vi "SEC code V4.9.vi"() -> ()   [LabVIEW 2022 SP3]
uses:
  SEC code V3.1/Drivers and Aux files/user.lib/atmcd32d.llb/Shutter_type typedef.ctl
  C:/Program Files/Metrohm Autolab/Autolab SDK 1.10/EcoChemie.Autolab.Sdk.dll
  Program Files/Metrohm Autolab/Autolab SDK 1.10/EcoChemie.Autolab.Sdk.dll
  SEC code V3.1/Drivers and Aux files/State.ctl
  SEC code V3.1/Drivers and Aux files/SECenumctl.ctl
  SEC code V3.1/Drivers and Aux files/user.lib/atmcd32d.llb/TriggerMode_mode typedef.ctl
  SEC code V3.1/Drivers and Aux files/OSSPEC.ctl
  SEC code V3.1/Drivers and Aux files/OSPEC-enum.ctl
  Labview/IVIUM/IVIUM_remdriver.lvlib
panel:
  out "POtential PD":dbl
  out "Current PD":dbl
  in  "Tab Control 5":enum32{"AUTOLAB", "IVIUM", "iDUS", "Kymera"}(tab)
  out "current":dbl
  out "Error after autolab connection?":errorcluster
  out "Autolab Connected?":bool
  out "Voltage":dbl
  out "PotentialOverload":bool
  out "Bandwidth":i32(ring) items=["UltraHigh_Speed", "High_Speed", "High_Stability"]
  out "CurrentRange":i32(ring) items=["CR07_1A"=0, "CR06_10A"=1, "CR01_100A"=2, "CR00_1000A"=3, "CR05_20A"=20, "CR04_40A"=40, "CR03_50A"=60, "CR02_80A"=80, "CR19_1pA"=-12, "CR18_10pA"=-11, "CR17_100pA"=-10, "CR16_1nA"=-9, "CR15_10nA"=-8, "CR14_100nA"=-7, "CR13_1uA"=-6, "CR12_10uA"=-5, "CR11_100uA"=-4, "CR10_1mA"=-3, "CR09_10mA"=-2, "CR08_100mA"=-1]
  out "Mode":i32(ring) items=["Potentiostatic", "Galvanostatic"]
  out "Measured voltage":dbl
  out "CurrentOverload":bool
  out "Cell on?":bool
  out "current":dbl caption="Current (A)" format="%_4g"
  out "cell on":bool
  out "V (during measurment)":dbl
  out "Potentiostat Status":string
  out "T reached?":bool
  out "Shut down sequence run?":bool
  out "Curent Temp":i32
  in  "Tab Control 4":T1(tab)
  in  "Use autolab?":bool=TRUE
  in  "Embedded Exe File":path=path "C:/Program Files/Metrohm Autolab/Autolab SDK 2.1/Hardware Setup Files/Adk.x"
  in  "Hardware Setup File":path=path "C:/ProgramData/Metrohm Autolab/13.0/HardwareSetup.AUT55157.xml"
  in  "Bandwidth 2":i32(ring)=2 items=["UltraHigh_Speed", "High_Speed", "High_Stability"]
  in  "Start potential (V)":dbl=0.2
  in  "Stop potential (V)":dbl=0.7
  in  "Increment (V)":dbl=0.05
  in  "Default Potential (V)":dbl=0.2
  in  "Wait before \nspectrum (s)":dbl=0.1
  in  "Equilibration \ntime (s)":u32=5
  in  "Reverse Scan\ndirection":bool
  in  "(update and read)":bool
  in  "Tab Control 3":T2(tab)
  in  "Inetegration Time (us)":i32=5000
  in  "Continuous \nStrobe Delay (us)":i32
  in  "Use iDus?":bool=TRUE
  in  "Return detector \nto room T?":bool
  in  "Init, Cool, read dark,\nOR\nWarm/de-init detector":bool
  in  "Temperature\n(degrees C)":i32=-80
  in  "Number of scans in kinetic cycle":i32=30
  in  "Exposure time (s)":dbl=0.03
  in  "Tab Control 2":T3(tab)
  in  "V 1 time (s)":dbl=10.0
  in  "V off time":dbl=30.0
  in  "Sampling delay (s)":dbl
  in  "V 2 time (s)":dbl=20.0
  in  "Run OSPSEC":bool
  in  "squre wave":bool
  out "OCP I (close to 0)":dbl
  out "OCP":dbl format="%_3f"
  in  "V1 (V)":dbl=0.4
  in  "V2 (V)":dbl=0.8
  in  "Slow sample time (s)":dbl=1500.0
  out "Time during PD":u32
  in  "File Name":string="test-1"
  in  "Path":path=path "C:/Data"
  in  "Tab Control":T4(tab)
  out "?":T5(graph)
  out "?":cluster{i32[], dbl[]}(graph)
  out "?":T5(graph)
  out "?":T5(graph)
  out "?":cluster{dbl[], dbl[]}(graph)
  out "?":cluster{i32[], "array":i32[]}(graph)
  out "I_overload":bool
  out "Aninput1_overload":bool
  out "E_overload":bool
  out "cell-off button pressed":bool
  in  "Default\nCurrent range":T6(ring)=enum."100 uA"
  in  "Default Filter":T7(ring)=enum."10 kHz"
  out "Device serial number":string
  in  "Set Stability":T8(ring)=enum."Standard"
  out "Number of Spectrometers":i32
  out "IDus not in read loop? (kinetic)":bool
  out "Get status return code":dbl
  out "xpixels":i32
  out "ypixels":i32
  out "Calculated exposure time":sgl format="%.2f"
  out "Check timings return code":u32
  out "Set temprature\nreturn code":u32
  out "get aquired data return code":u32
  out "Start Aquisition return code":u32
  out "Init. return code":u32
  out "Cooler Off return code":u32
  out "Time before the start of current aquisition (ms)":u32
  out "Time  after the aquisition (before fetch data), (ms)":u32
  in  "Shutter opens on TTL":T9=enum."TTL High"
  in  "Shutter open and close time":i32
  out "Get aqisition ok? (kinetic mode)":bool
  out "Time taken to apply V2":u32
  out "Values to re-intialise to at end\nof the measument":T10
  out "V2 applied?":bool
  out "ContinuousStrobe Out":u32
  out "Wrapper Out":u32
  out "WL Values":dbl[](array[numeric])
  out "Adc":refnum<k24>
  out "Sampler 2":refnum<k24>
  out "Dio":refnum<k24>
  out "Dac":refnum<k24>
  out "instrument":refnum<k24>
  out "Ei":refnum<k24>
  out "AutolabConnection":refnum<k24>
  out "EI status supported for":string[](array[string])
  out "TemperatureOverload":bool
  out "ManualCellSwitch":bool
  out "Oscillation":bool
  in  "Exit and disconnect":bool
  # "Checklist for avoiding errors:\n(1) Light on the IVIUM should be blue with red flashes\nIf the system crahes and the light is red then connect and disconnect in IVUM soft/turn stat off/on\n(2) Maya Pro should read in ocean view/or the get intensity program\nIf maya is not reading connect and disconnect USB\n(3) If errors persist rrepeat steps 1 + 2 then re-compile code by clicking the\nwhite (run) whilst holding down CRTL + (left) SHIFT\n(4) At the end of a potential decay measurment click exit before starting a new measurment\n(5) IF USING THE iDus DO NOT EXIT WITHOUT WARMING CAMERA BACK TO ROOM T,YOU \nWILL DAMAGE IT \n(6) if the IVIUM.dll does not load click broken arrows and \"show error\" until you see the call library function (see blue circles). Double click on this and paste the following into the directory (red circle):   \n%windir%\\Labview\\IVIUM\\IVIUM_remdriver.dll"
  # "Program control"
  # "Potential decay control"
  # "Spectrometer control"
  # "System status"
  # "SEC control"
  # "Cell on?"
  # "Use the integration time program in the same folder as this program\nto get the optimum value. For kinetic mode the time resolution is limited \nby integration time"
  # "Unless you know what you are doing keep these at 0.03 and 30"
  # "I overload overload"
  # "off button pressed"
  # "Aninput1 overload"
  # "E overload"
  # "OSPEC loop exit"
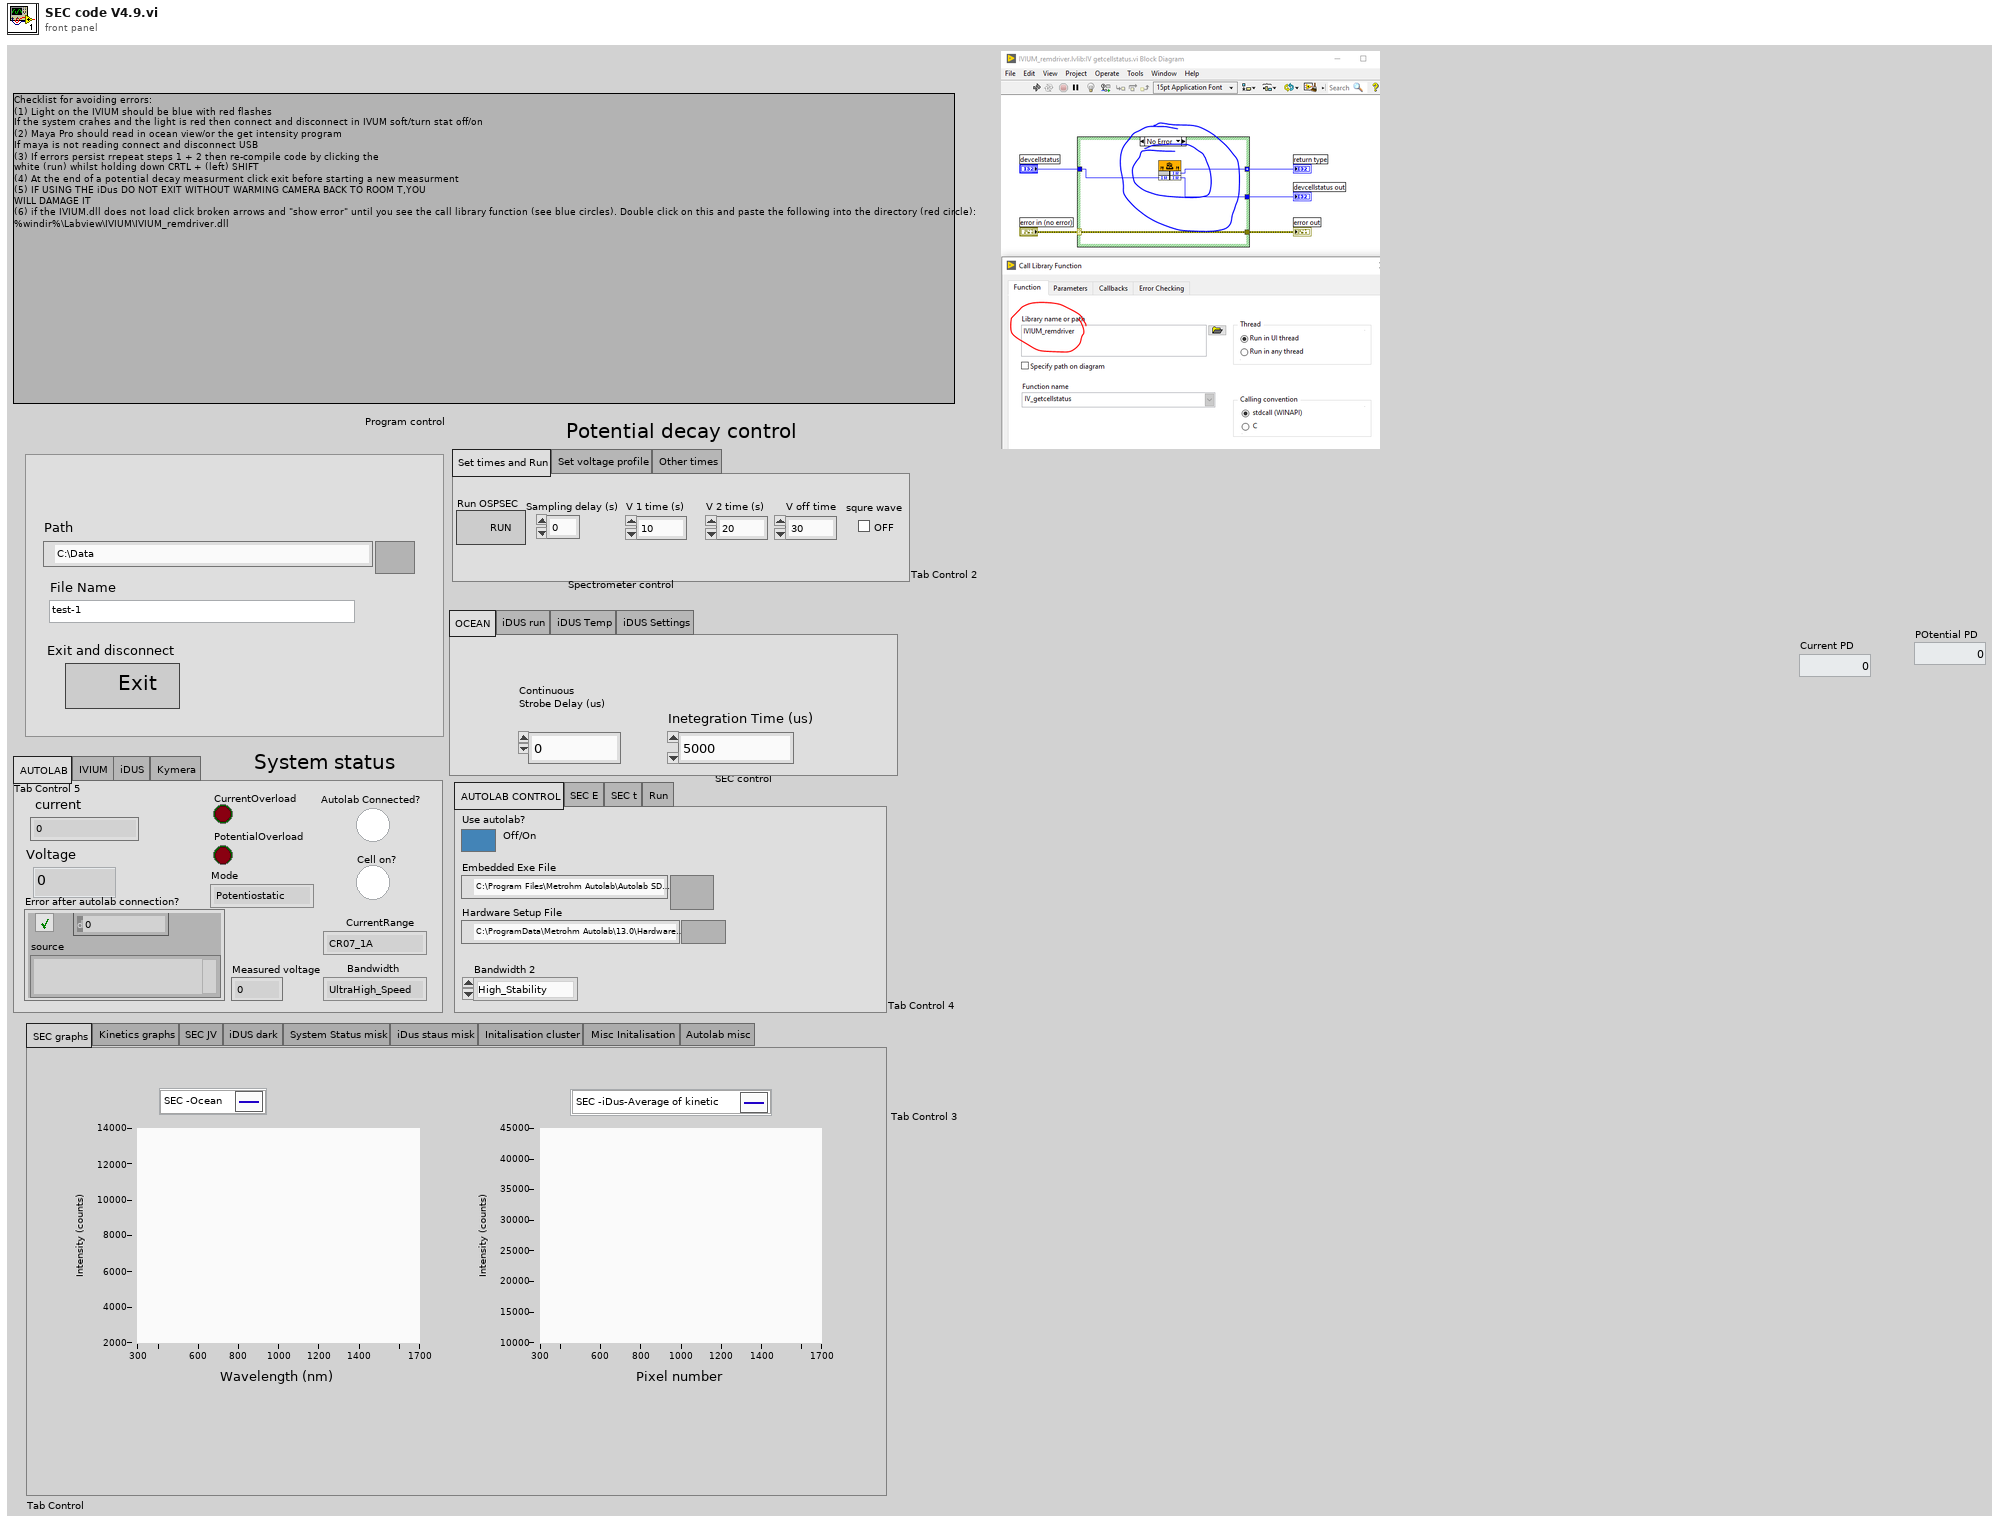
[diagram p1: front panel]
types:
  T1 = enum32{"AUTOLAB CONTROL", "SEC E", "SEC t", "Run"}
  T2 = enum32{"OCEAN", "iDUS run", "iDUS Temp", "iDUS Settings"}
  T3 = enum32{"Set times and Run", "Set voltage profile", "Other times"}
  T4 = enum32{"SEC graphs", "Kinetics graphs", "SEC JV", "iDUS dark", "System Status misk", "iDus staus misk", "Initalisation cluster", "Misc Initalisation ", "Autolab misc"}
  T5 = cluster{"WL Values":dbl[], "Spectrum Values":dbl[]}
  T6 = enum16{"10 A", "1 A", "100 mA", "10 mA", "1 mA", "100 uA", "10 uA", "1 uA", "100 nA", "10 nA", "1 nA", "100 pA", "10 pA", "1 pA"}
  T7 = enum16{"1 MHz", "100 kHz", "10 kHz", "1 kHz", "10 Hz"}
  T8 = enum16{"High Speed", "Standard", "High Stability"}
  T9 = typedef "Shutter_type typedef.ctl" = enum16{"TTL Low", "TTL High"}
  T10 = cluster{"Currents":dbl[], "Potentials":dbl[], "Device Status":string, "Device serial no":string, "Current":dbl, "Default \nPotential":dbl, "I overload":bool, "Cell On":bool, "E overload":bool, "Aninput1 overload":bool, "Cell off button pressed":bool, "Start potential":dbl, "Stop potential":dbl, "Increment":dbl, "SEC":dbl[], "Path":path, "File name":string}
  T11 = cluster{"Current array":dbl[], "Potential array":dbl[], "Status":string, "Serial No":string, "Current":dbl, "Default\n potential":dbl, "I overload":bool, "Cell on":bool, "E overload":bool, "Cell of button pressed":bool, "Aninput1 overload":bool, "Stop \npotential":dbl, "Start \npotential":dbl, "Increment":dbl, "Spectrum":dbl[][], "Path":path, "File Name":string, "Sample rate":dbl, "V2 time":dbl, "V off time":dbl, "V 2":dbl, "V 1":dbl, "V1 time":dbl, "Time array":dbl[], "Integration time":i32, "Continous strobe delay":i32, "Time elapsed ":i32, "Start time":i32, "Time for E measurment":i32[], "Time for I measurment ":i32[], "Time for spectrum measurment":i32[], "Return detector to \nroom T":bool, "Number of scans in kinetic cycle":i32, "Exposure time":i32}
  T12 = typedef "State.ctl" = enum16{"Initialize", "Wait for Event", "Run SEC", "Run OSPEC", "Initialse and cool iDus", "Exit"}
  T13 = typedef "SECenumctl.ctl" = enum16{"Read spectrum from Ocean", "Read spectrum from iDus", "Apply potential", "Wait", "Apply potential Autolab"}
  T14 = typedef "TriggerMode_mode typedef.ctl" = enum16{"Internal", "External", "N/A (2)", "N/A (3)", "N/A (4)", "N/A (5)", "External Start", "External Exposure (Bulb)", "N/A (8)", "External FVB EM", "Software", "N/A (11)", "External Charge Shifting"}
  T15 = typedef "OSSPEC.ctl" = enum16{"Read Potential and spectrum", "Read current and spectrum", "Reinitialise Cell", "Apply V1", "End measurment", "Apply V2"}
  T16 = typedef "OSPEC-enum.ctl" = enum16{"Check exit", "Read", "Wait"}
  T17 = enum16{"off", "EStat4EL", "EStat2EL", "EStatDummy1", "EStatDummy2", "EStatDummy3", "EStatDummy4", "IStat4EL", "IStat2EL", "IStatDummy", "BiStat4EL", "BiStat2EL"}
  T18 = typedef "Error Code Enum typedef.ctl" = enum32{"N/A (0)", "DRV_ERROR_CODES", "DRV_SUCCESS", "DRV_VXDNOTINSTALLED", "DRV_ERROR_SCAN", "DRV_ERROR_CHECK_SUM", "DRV_ERROR_FILELOAD", "DRV_UNKNOWN_FUNC", "DRV_ERROR_VXD_INIT", "DRV_ERROR_ADDRESS", "DRV_ERROR_PAGELOCK", "DRV_ERROR_PAGEUNLOCK", "DRV_ERROR_BOARDTEST", "DRV_ERROR_ACK", "DRV_ERROR_UP_FIFO", "DRV_ERROR_PATTERN", "N/A (16)", "DRV_ACQUISITION_ERRORS", "DRV_ACQ_BUFFER", "DRV_ACQ_DOWNFIFO_FULL", "DRV_PROC_UNKONWN_INSTRUCTION", "DRV_ILLEGAL_OP_CODE", "DRV_KINETIC_TIME_NOT_MET", "DRV_ACCUM_TIME_NOT_MET", "DRV_NO_NEW_DATA", "N/A (25)", "DRV_SPOOLERROR", "N/A (27)", "N/A (28)", "N/A (29)", "N/A (30)", "N/A (31)", "N/A (32)", "DRV_TEMPERATURE_CODES", "DRV_TEMPERATURE_OFF", "DRV_TEMPERATURE_NOT_STABILIZED", "DRV_TEMPERATURE_STABILIZED", "DRV_TEMPERATURE_NOT_REACHED", "DRV_TEMPERATURE_OUT_RANGE", "DRV_TEMPERATURE_NOT_SUPPORTED", "DRV_TEMPERATURE_DRIFT", "N/A (41)", "N/A (42)", "N/A (43)", "N/A (44)", "N/A (45)", "N/A (46)", "N/A (47)", "N/A (48)", "DRV_GENERAL_ERRORS", "DRV_INVALID_AUX", "DRV_COF_NOTLOADED", "DRV_FPGAPROG", "DRV_FLEXERROR", "DRV_GPIBERROR", "N/A (55)", "N/A (56)", "N/A (57)", "N/A (58)", "N/A (59)", "N/A (60)", "N/A (61)", "N/A (62)", "N/A (63)", "DRV_DATATYPE", "DRV_DRIVER_ERRORS", "DRV_P1INVALID", "DRV_P2INVALID", "DRV_P3INVALID", "DRV_P4INVALID", "DRV_INIERROR", "DRV_COFERROR", "DRV_ACQUIRING", "DRV_IDLE", "DRV_TEMPCYCLE", "DRV_NOT_INITIALIZED", "DRV_P5INVALID", "DRV_P6INVALID", "DRV_INVALID_MODE", "DRV_INVALID_FILTER", "DRV_I2CERRORS", "DRV_I2CDEVNOTFOUND", "DRV_I2CTIMEOUT", "DRV_P7INVALID", "N/A (84)", "N/A (85)", "N/A (86)", "N/A (87)", "N/A (88)", "N/A (89)", "DRV_IOCERROR", "DRV_VRMVERSIONERROR"}
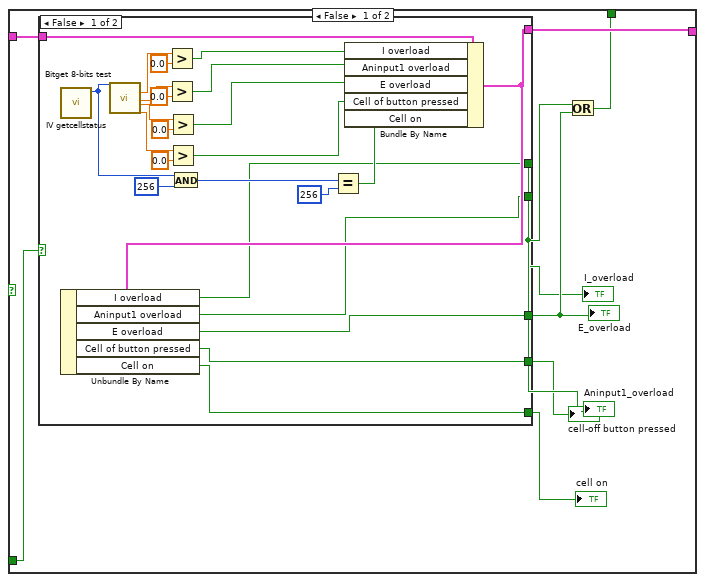
[diagram p2: hidden frame]
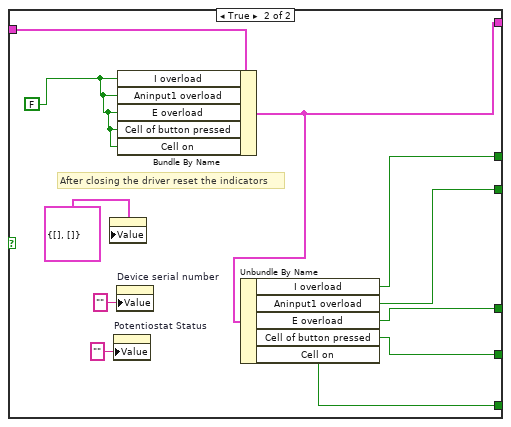
[diagram p3: hidden frame]
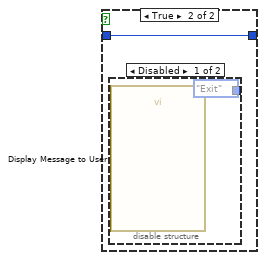
[diagram p4: hidden frame]
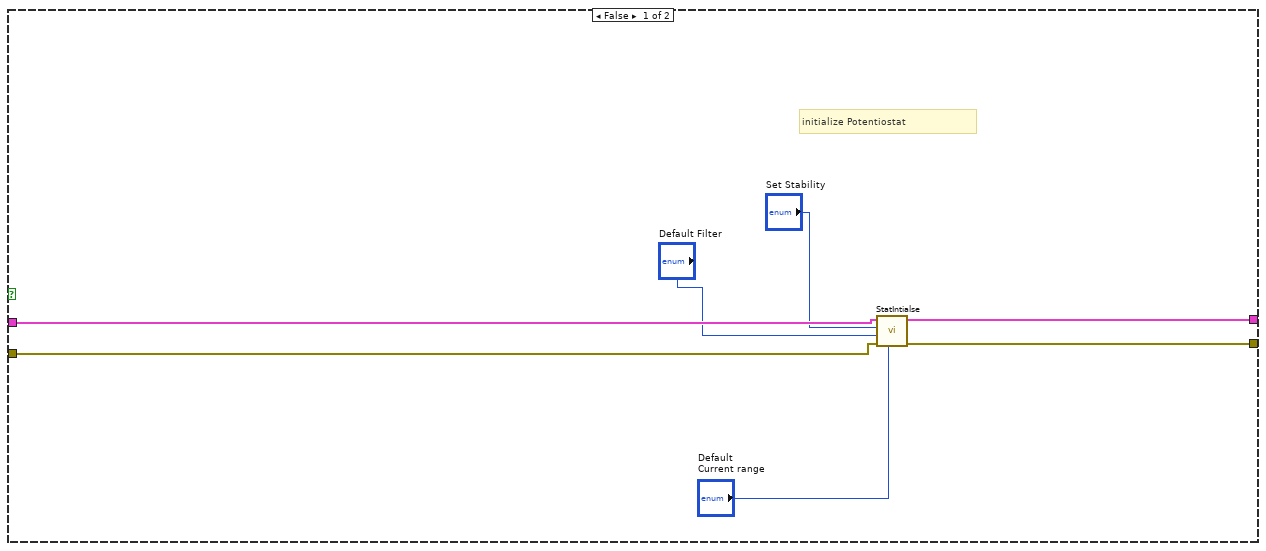
[diagram p6: hidden frame]
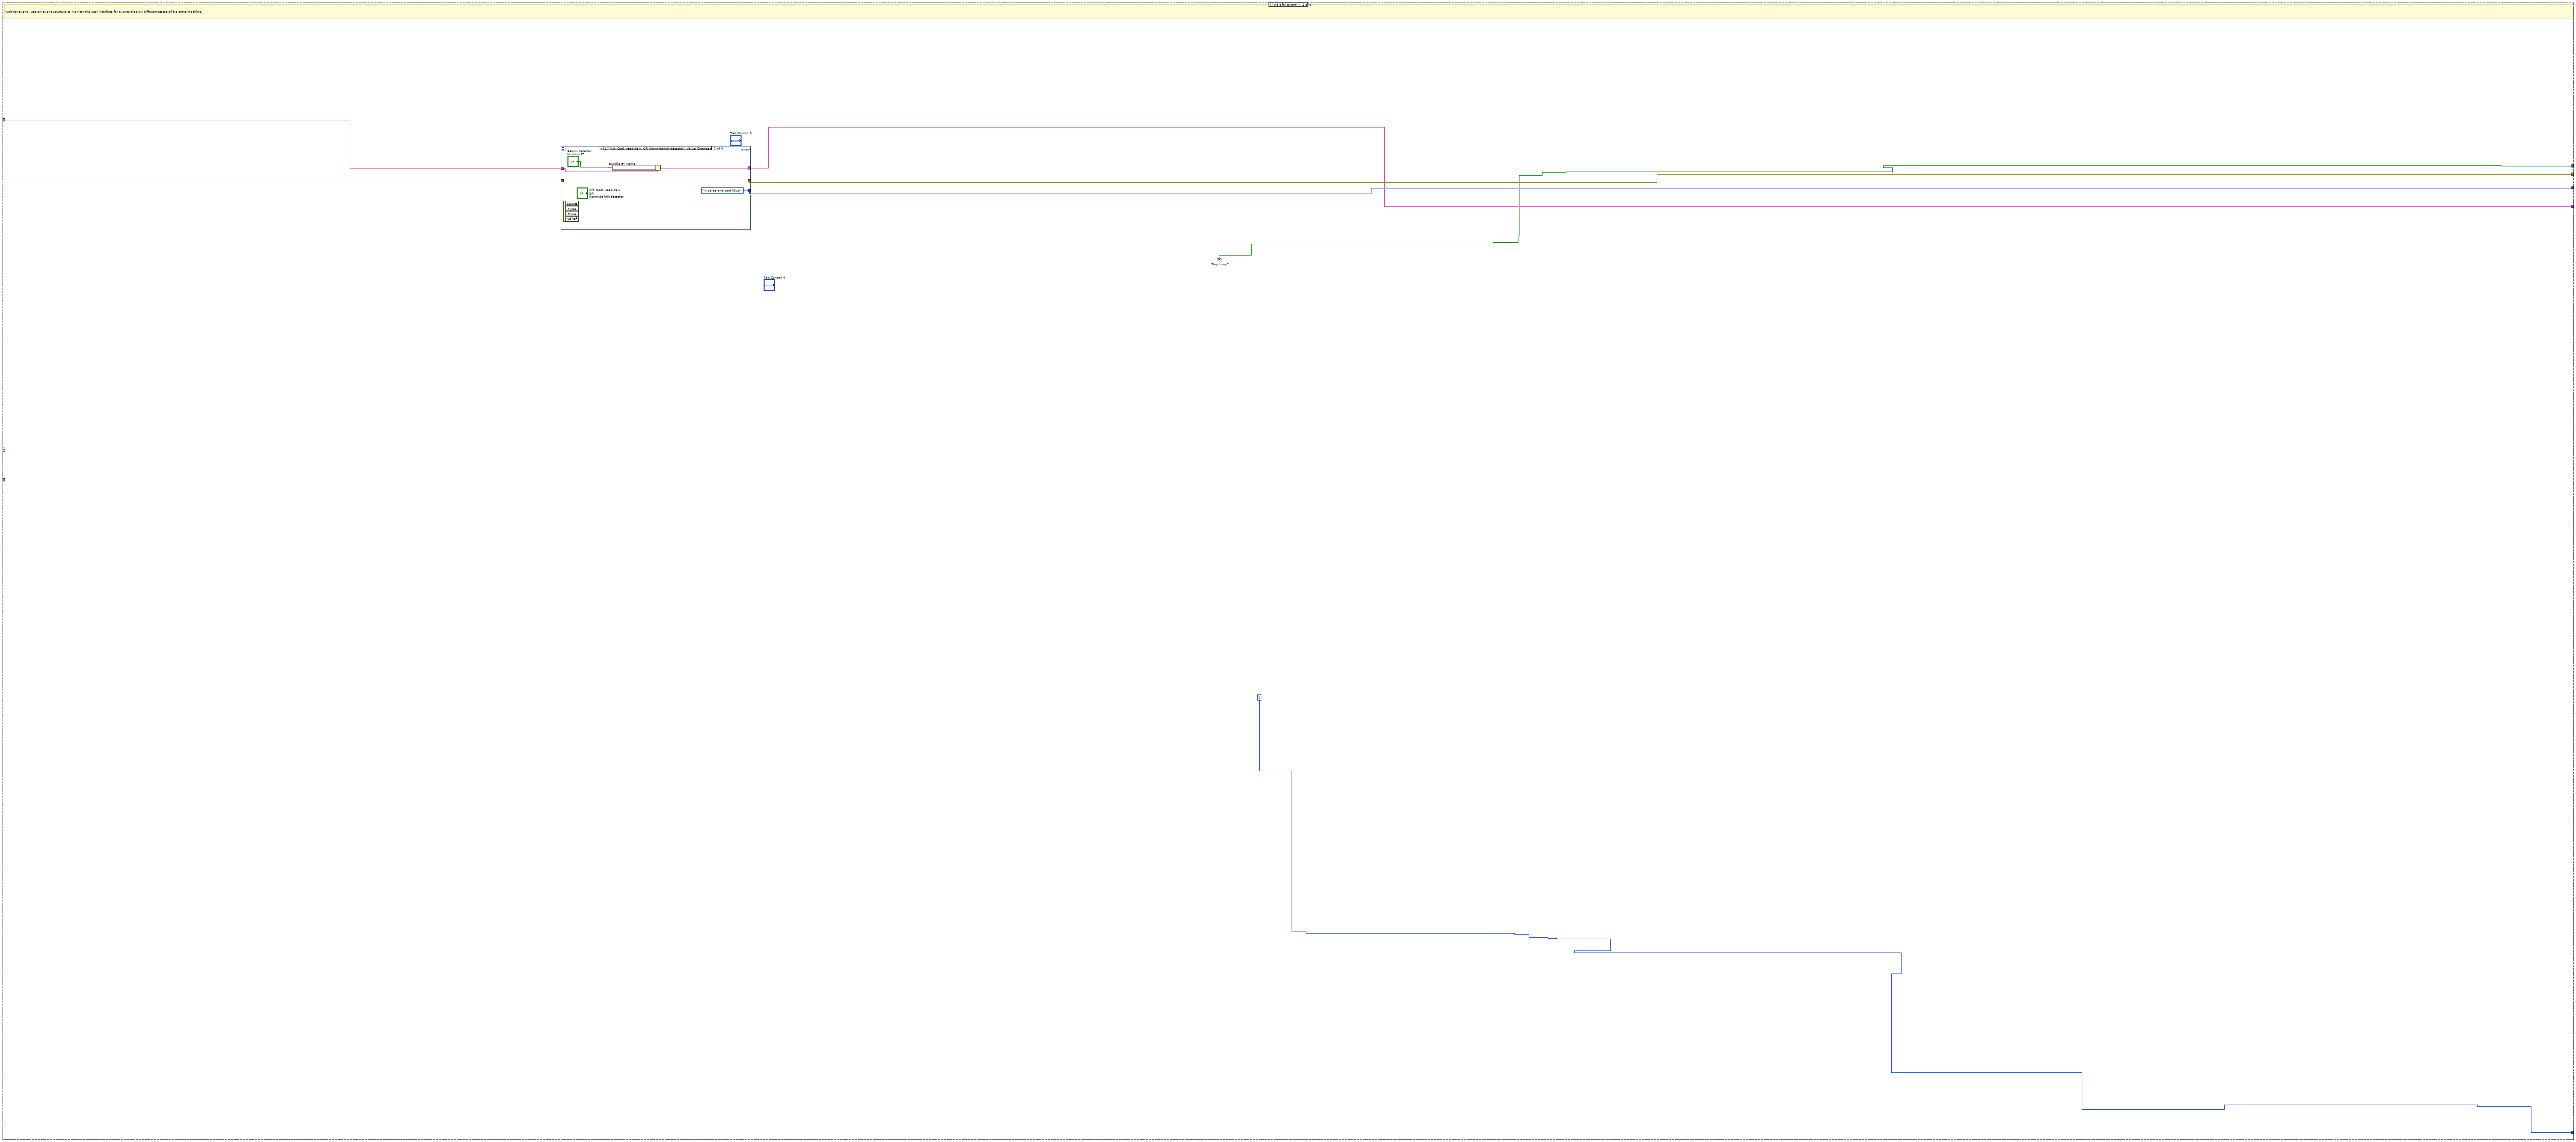
[diagram p7: hidden frame]
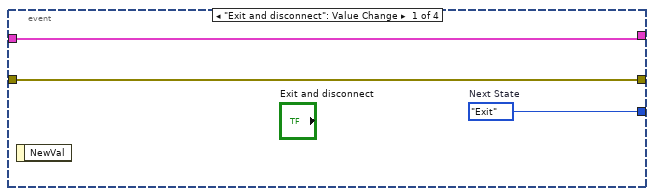
[diagram p8: hidden frame]
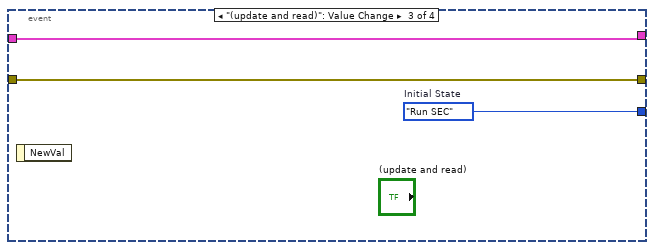
[diagram p9: hidden frame]
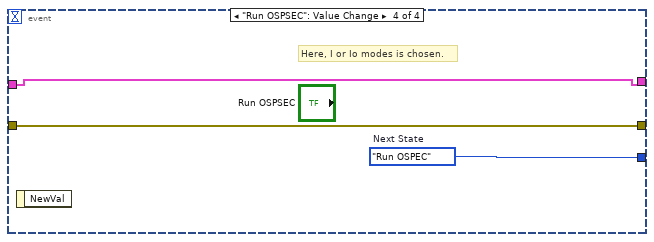
[diagram p10: hidden frame]
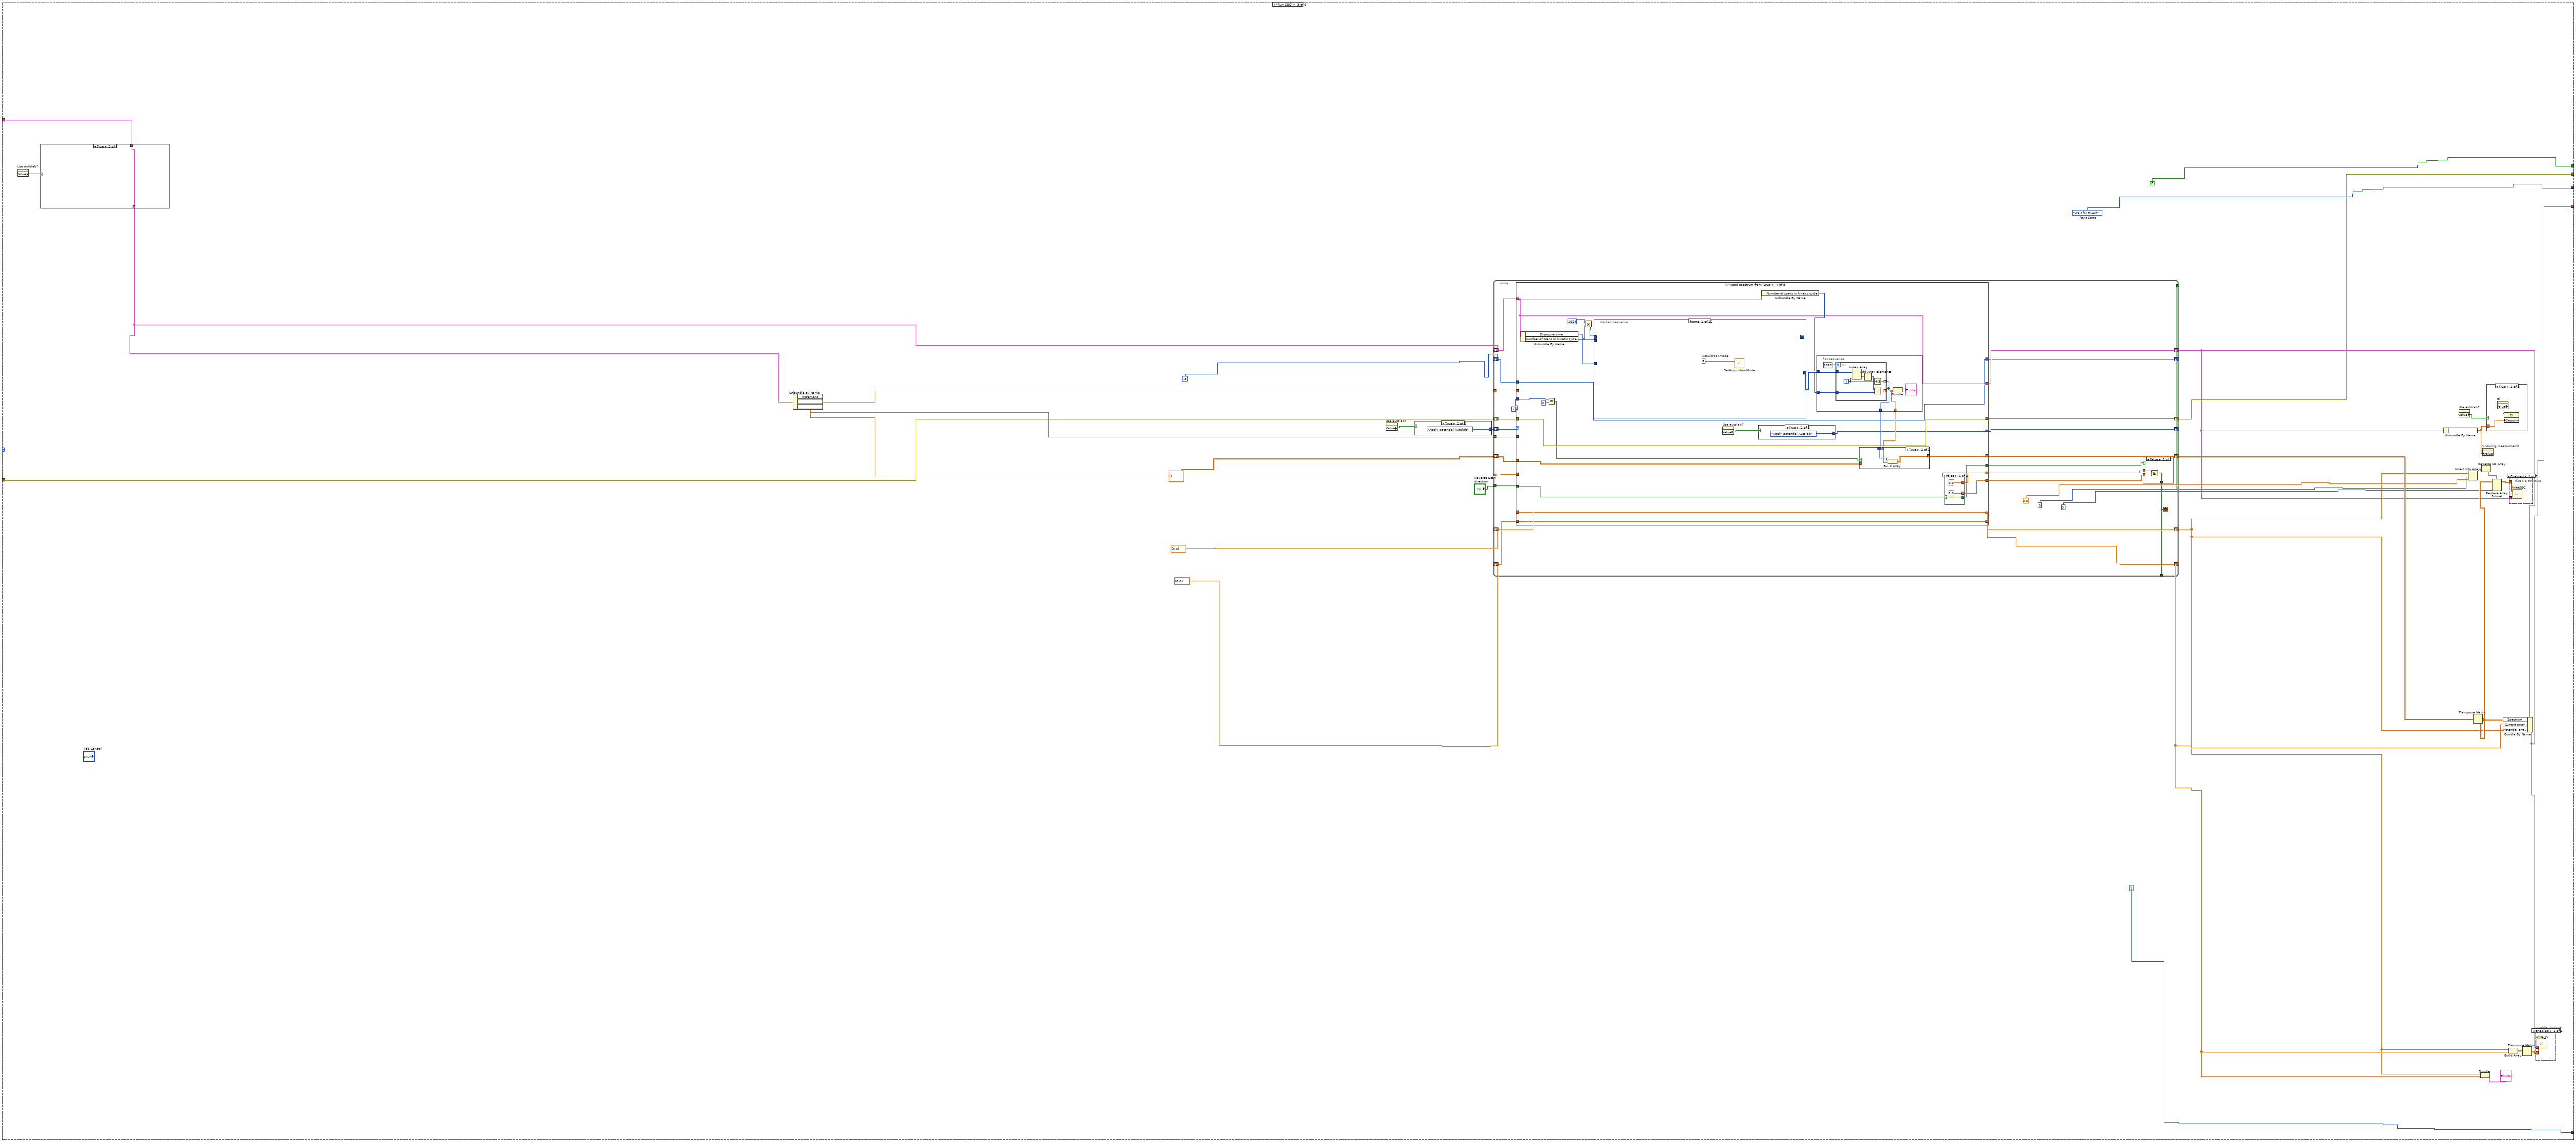
[diagram p11: hidden frame]
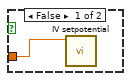
[diagram p12: hidden frame]
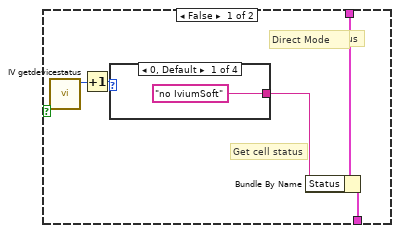
[diagram p13: hidden frame]
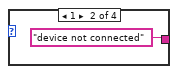
[diagram p14: hidden frame]
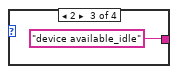
[diagram p15: hidden frame]
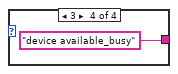
[diagram p16: hidden frame]
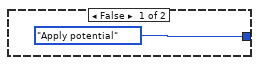
[diagram p17: hidden frame]
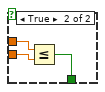
[diagram p20: hidden frame]
diagram:
  w1 = T11 {"Current array"=[], "Potential array"=[], "Status"="", "Serial No"="", "Current"=0.0, "Default\n potential"=0.0, "I overload"=FALSE, "Cell on"=FALSE, "E overload"=FALSE, "Cell of button pressed"=FALSE, "Aninput1 overload"=FALSE, "Stop \npotential"=0.0, "Start \npotential"=0.0, "Increment"=0.0, "Spectrum"=[], "Path"=path "", "File Name"="", "Sample rate"=0.0, "V2 time"=0.0, "V off time"=0.0, "V 2"=0.0, "V 1"=0.0, "V1 time"=0.0, "Time array"=[], "Integration time"=0, "Continous strobe delay"=0, "Time elapsed "=0, "Start time"=0, "Time for E measurment"=[], "Time for I measurment "=[], "Time for spectrum measurment"=[], "Return detector to \nroom T"=FALSE, "Number of scans in kinetic cycle"=0, "Exposure time"=0}  # Init cluster
  w3 = State."Initialize"  # Initial State
  n1 = while {
    shift-right: [w21] -> _
    shift-left: w3 -> [w38]
    shift-right: [w24] -> _
    shift-left: w1 -> [w17]
    shift-right: [w25] -> _
    shift-left: errorcluster {"status"=FALSE, "code"=0, "source"=""} ("error constant") -> [w37]
    stop <- w35 stop-if-true
    # "Main VI State Machine"
    n2 = Bundle By Name(cluster=w17, "Sample rate"="Sampling delay (s)", "V1 time"="V 1 time (s)", "V2 time"="V 2 time (s)", "V off time"="V off time", "V 2"="V2 (V)", "V 1"="V1 (V)", "Integration time"="Inetegration Time (us)", "Continous strobe delay"="Continuous \nStrobe Delay (us)", "Exposure time"="Exposure time (s)", "Number of scans in kinetic cycle"="Number of scans in kinetic cycle") -> (w11:T11)
    n3 = Bundle By Name(cluster=w11, "Default\n potential"="Default Potential (V)", "Start \npotential"="Start potential (V)", "Stop \npotential"="Stop potential (V)", "Increment"="Increment (V)", "Path"="Path", "File Name"="File Name") -> (w23:T11)
    n4 = case shown="\"Initialize\"" w38 {
      tunnel: [w94 w137 w185 w490 State."Wait for Event" ("f") w1602] -> w7
      tunnel: [w93 w134 FALSE ("Stop Loop?") w487 FALSE ("Stop Loop?") _] -> w36
      tunnel: w23 -> [w91 w131 w174 w491 w528 w1600]
      tunnel: [w90 w132 w158 w491 w524 w1600] -> w31
      tunnel: w37 -> [w95 w136 w183 w493 w526 w1599]
      tunnel: [w96 w135 w182 w494 w525 w1599] -> w25
      tunnel: [1 ("devconnect") 1 ("devconnect") 1 ("devconnect") w492 1 ("devconnect") 1 ("devconnect")] -> w22
      frame "Initialize" {
        w93 = FALSE  # Stop Loop?
        w94 = State."Wait for Event"  # Next State
        # "Initialize - Initialize variables needed"
        n5 = case shown="True" "Use autolab?" {
          tunnel: [w104 w108] -> w96
          tunnel: w95 -> [w103 _]
          tunnel: w91 -> [w102 w130]
          tunnel: [w98 w130] -> w90
          frame False {
            # "initialize Potentiostat"
            n6 = call "StatIntialse.vi"("Init cluster 2"=w102, "Set Stability"="Set Stability", "Default\n Filter"="Default Filter", "error in (no error)"=w103, "Default\nCurrent range"="Default\nCurrent range") -> ("Init cluster"=w98:T11, "error out"=w104:errorcluster)  [unwired: 4 in]
          }
          frame True {
            w111 = 0 items=["Potentiostatic", "Galvanostatic"] ("Mode")
            w112 = -3 items=["CR07_1A"=0, "CR06_10A"=1, "CR01_100A"=2, "CR00_1000A"=3, "CR05_20A"=20, "CR04_40A"=40, "CR03_50A"=60, "CR02_80A"=80, "CR19_1pA"=-12, "CR18_10pA"=-11, "CR17_100pA"=-10, "CR16_1nA"=-9, "CR15_10nA"=-8, "CR14_100nA"=-7, "CR13_1uA"=-6, "CR12_10uA"=-5, "CR11_100uA"=-4, "CR10_1mA"=-3, "CR09_10mA"=-2, "CR08_100mA"=-1] ("CurrentRange")
            w114 = 1 items=["Off", "On"] ("CellOnOff")
            n7 = call "Connect AutoLab.vi"("Embedded Exe File"="Embedded Exe File", "Hardware Setup File"="Hardware Setup File") -> ("error out"=w119:errorcluster, ".NET Refnum out"=w128:refnum<k24>)  [unwired: 8 in]
            "Error after autolab connection?" <- w119
            n8 = property class="Instrument"(reference=w128, error in=w119) -> (reference out=→"instrument":refnum<k24>, error out=w120:errorcluster, "Adc"=→"Adc":refnum<k24>, "Dac"=→"Dac":refnum<k24>, "Dio"=→"Dio":refnum<k24>, "AutolabConnection"=w116:refnum<k24>, "Ei"=w107:refnum<k24>)
            "AutolabConnection" <- w116
            n9 = property class="AutolabConnection"(reference=w116) -> ("IsConnected"=→"Autolab Connected?":bool)  [unwired: 1 in, 2 out]
            n10 = property class="EI"(reference=w107, error in=w120) -> (reference out=→"Ei":refnum<k24>, error out=w127:errorcluster, "Sampler"=→"Sampler 2":refnum<k24>)
            n11 = property on="Bandwidth 2" class="Ring (strict)"() -> ("Value"=w113:i32)  [unwired: 2 in, 2 out]
            n12 = property on="Default Potential (V)" class="DigNum (strict)"() -> ("Value"=w110:dbl)  [unwired: 2 in, 2 out]
            n13 = Build Array(w120, w127) -> (w121:errorcluster[])
            n14 = Merge Errors(w121) -> (w109:errorcluster)
            n15 = property class="EI"(reference=w107, error in=w109, "Bandwidth"=w113, "CellOnOff"=w114, "CurrentRange"=w112, "Mode"=w111, "Setpoint"=w110) -> (error out=w108:errorcluster, "Current"=w106:dbl, "Potential"=w105:dbl)  [unwired: 1 out]
            n16 = property on="current" class="DigNum (strict)"("Value"=w106) -> ()  [unwired: 2 in, 2 out]
            n17 = property on="Voltage" class="DigNum (strict)"("Value"=w105) -> ()  [unwired: 2 in, 2 out]
          }
        }
        n18 = property on="V2 applied?" class="Bool (strict)"("Value"=FALSE ("V2 applied")) -> ()  [unwired: 2 in, 2 out]
        "Values to re-intialise to at end\nof the measument" <- T10 {"Currents"=[], "Potentials"=[], "Device Status"="", "Device serial no"="", "Current"=0.0, "Default \nPotential"=0.0, "I overload"=FALSE, "Cell On"=FALSE, "E overload"=FALSE, "Aninput1 overload"=FALSE, "Cell off button pressed"=FALSE, "Start potential"=0.0, "Stop potential"=0.0, "Increment"=0.0, "SEC"=[], "Path"=path "", "File name"=""} ("Values to re-intialise to at end\nof the measument")
      }
      frame "Wait for Event" {
        w134 = FALSE  # Stop Loop?
        # "Wait for Event - Use an Event Structure to monitor the user interface for events that run different states of the state machine."
        n19 = event shown="[1] \"Init, Cool, read dark, OR Warm/de-init detector\": Value Change" {
          selector: _ -> [_ _ _ _]
          dyn-events: _ -> [_ _ _ _]
          timeout: _ -> [_ _ _ _]
          tunnel: [w140 State."Initialse and cool iDus" ("Next State") w147 w151] -> w137
          tunnel: w136 -> [w139 w145 w148 w150]
          tunnel: [w139 w145 w148 w150] -> w135
          tunnel: w131 -> [w138 w143 w146 w149]
          tunnel: [w138 w141 w146 w149] -> w132
          event "Exit and disconnect": Value Change {
            w140 = State."Exit"  # Next State
            n20 = event-data() -> ()  [unwired: 1 in, 1 out]
          }
          event "Init, Cool, read dark,\nOR\nWarm/de-init detector": Value Change {
            n21 = event-data() -> ()  [unwired: 1 in, 4 out]
            n22 = Bundle By Name(cluster=w143, "Return detector to \nroom T"="Return detector \nto room T?") -> (w141:T11)
          }
          event "(update and read)": Value Change {
            w147 = State."Run SEC"  # Initial State
            n23 = event-data() -> ()  [unwired: 1 in, 1 out]
          }
          event "Run OSPSEC": Value Change {
            w151 = State."Run OSPEC"  # Next State
            # "Here, I or Io modes is chosen."
            n24 = event-data() -> ()  [unwired: 1 in, 1 out]
          }
        }
      }
      frame "Run SEC" {
        w185 = State."Wait for Event"  # Next State
        n25 = property on="Use autolab?" class="Bool (strict)"() -> ("Value"=w153:bool)  [unwired: 2 in, 2 out]
        n26 = case shown="True" w153 {
          tunnel: w174 -> [w191 w199]
          tunnel: [w190 w199] -> w160
          frame False {
            # "Get cell status"
            # "Get Device Status"
            # "Direct Mode"
            n27 = call "IV getdevicestatus.vi"() -> ("return type"=w193:i32)  [unwired: 10 in, 1 out]
            n28 = Increment(x=w193) -> (x+1=w192:i32)
            n29 = case shown="0, Default" w192 {
              tunnel: ["no IviumSoft" "device not connected" "device available_idle" "device available_busy"] -> w194
              frame 0, Default {
              }
              frame 1 {
              }
              frame 2 {
              }
              frame 3 {
              }
            }
            n30 = Bundle By Name(cluster=w191, "Status"=w194) -> (w190:T11)
          }
          frame True {
          }
        }
        n31 = Unbundle By Name(w160) -> ("Increment"=w180:dbl, "Start \npotential"=w184:dbl, "Stop \npotential"=w175:dbl)
        n32 = property on="Use autolab?" class="Bool (strict)"() -> ("Value"=w155:bool)  [unwired: 2 in, 2 out]
        n33 = case shown="True" w155 {
          tunnel: [SECenumctl."Apply potential" SECenumctl."Apply potential Autolab"] -> w181
          frame False {
          }
          frame True {
          }
        }
        n34 = while {
          shift-right: [w227] -> w157
          shift-left: w160 -> [w228]
          tunnel: w180 -> [w223]
          tunnel: w184 -> [w222]
          shift-right: [w224] -> w182
          shift-left: w183 -> [w225]
          shift-right: [w216] -> _
          shift-left: w181 -> [w220]
          shift-right: [w218] -> w159
          shift-left: dbl[] [0.0] -> [w217]
          shift-right: [w213] -> w163
          shift-left: dbl[] [0.0] -> [w214]
          tunnel: w175 -> [w215]
          shift-right: [w212] -> w173
          shift-left: dbl[][] [] -> [w211]
          tunnel: "Reverse Scan\ndirection" -> [w210]
          tunnel: [w208] -> _
          tunnel: [w208] -> _
          shift-right: [w207] -> _
          shift-left: -3 ("y") -> [w206]
          i -> [w226]
          stop <- w208 stop-if-true
          n35 = case shown="\"Read spectrum from iDus\"" w220 {
            tunnel: w228 -> [w251 w315 w350 w365 w459]
            tunnel: [w250 w314 w350 w365 w459] -> w227
            tunnel: w226 -> [w264 w324 _ w372 w468]
            tunnel: w225 -> [w261 w306 w346 w374 w469]
            tunnel: [w252 w295 w346 w374 w469] -> w224
            tunnel: w223 -> [w247 w312 _ _ _]
            tunnel: w222 -> [w263 w323 _ _ _]
            tunnel: [w244 w307 w349 w378 w474] -> w221
            tunnel: [w236 w310 w348 w377 w473] -> w219
            tunnel: [w255 w318 w347 w379 w472] -> w218
            tunnel: w217 -> [w256 w319 w347 w379 w472]
            tunnel: [SECenumctl."Wait" SECenumctl."Wait" w351 w360 w455] -> w216
            tunnel: w215 -> [w236 w310 _ _ _]
            tunnel: w214 -> [w254 w317 w342 w380 w470]
            tunnel: [w253 w316 w342 w380 w470] -> w213
            tunnel: [w248 w313 w341 w368 w462] -> w212
            tunnel: w211 -> [w248 w313 w341 w369 w461]
            tunnel: w210 -> [w237 w311 w340 w376 w460]
            tunnel: [w237 w311 w339 w375 w460] -> w209
            tunnel: w206 -> [w235 w305 w337 w362 w456]
            tunnel: [w235 w304 w337 w362 w456] -> w207
            frame "Apply potential", Default {
              # "Here, the while loop iterates three times for every one change of potential. The loop counter is therefore diveded by three, multipled by the increment and then added to the start  potential to give the next potential in the LSV. Potential is applied, then current is read. These go into a build array function . A wait is inclided to alow the sample to equilibriate at the start potential"
              n36 = Divide(x=w264, y=3) -> (x/y=w259:dbl)
              n37 = Multiply(x=w247, y=w259) -> (x*y=w262:dbl)
              n38 = Add(x=w262, y=w263) -> (x+y=w244:dbl)
              "V (during measurment)" <- w244
              n39 = call "IV setpotential.vi"("error in (no error)"=w261, "value"=w244) -> ("error out"=w258:errorcluster)  [unwired: 7 in, 2 out]
              n40 = Equal To 0?(x=w259) -> (x = 0?=w260:bool)
              n41 = case shown="True" w260 {
                tunnel: w258 -> [w274 w276]
                tunnel: [w274 w276] -> w257
                frame False {
                }
                frame True {
                  n42 = Multiply(x=u32 1000, y="Equilibration \ntime (s)") -> (x*y=w275:u32)
                  n43 = Wait (ms)(milliseconds to wait=w275) -> ()  [unwired: 1 out]
                }
              }
              n44 = Equal To 0?(x=w247) -> (x = 0?=w242:bool)
              n45 = Absolute Value(x=w244) -> (abs(x)=w245:dbl)
              n46 = Build Array (concatenate)(w244, w256) -> (w255:dbl[])
              n47 = Greater?(x=w245, y=3.0) -> (0:w243:bool)
              n48 = call "IV getcurrent.vi"("error in (no error)"=w257) -> ("error out"=w240:errorcluster, "value out"=w238:dbl)  [unwired: 8 in, 1 out]
              n49 = Or(x=w242, y=w243) -> (x .or. y?=w241:bool)
              n50 = flat-sequence {
                tunnel: w240 -> [w268]
                tunnel: [w268] -> w239
                tunnel: w238 -> [w267]
                frame #0 {
                  n51 = call "Current ranging routine (SubVI).vi"("Current"=w267) -> ()  [unwired: 11 in]
                  n52 = Wait (ms)(milliseconds to wait=u32 100) -> ()  [unwired: 1 out]
                }
              }
              n53 = case shown="True" w241 {
                frame False {
                }
                frame True {
                  # "abort if E >3 V or\ndelta E =0"
                  n54 = call "IV setcellon.vi"("cellon"=0) -> ("error out"=w272:errorcluster)  [unwired: 8 in, 2 out]
                  n55 = call "IV close.vi"("error in (no error)"=w272) -> ("error out"=w270:errorcluster)  [unwired: 9 in, 1 out]
                  n56 = call "Display Message to User2"("error in (no error)"=w270) -> ("OK"=w273:bool)  [unwired: 9 in, 1 out]
                  n57 = Stop(stop? (T)=w273) -> ()
                }
              }
              n58 = call "IV getcurrent.vi"("error in (no error)"=w239) -> ("error out"=w252:errorcluster, "value out"=w249:dbl)  [unwired: 8 in, 1 out]
              n59 = Bundle By Name(cluster=w251, "Current"=w249) -> (w250:T11)
              n60 = property on="current" class="DigNum (strict)"("Value"=w249) -> ()  [unwired: 2 in, 2 out]
              n61 = Build Array (concatenate)(w249, w254) -> (w253:dbl[])
            }
            frame "Apply potential Autolab" {
              w308 = 1 items=["Off", "On"] ("CellOnOff")
              w303 = 0 items=["Potentiostatic", "Galvanostatic"] ("Mode")
              # "Here, the while loop iterates three times for every one change of potential. The loop counter is therefore diveded by three, multipled by the increment and then added to the start  potential to give the next potential in the LSV. Potential is applied, then current is read. These go into a build array function . A wait is inclided to alow the sample to equilibriate at the start potential"
              n62 = Divide(x=w324, y=3) -> (x/y=w320:dbl)
              n63 = Multiply(x=w312, y=w320) -> (x*y=w322:dbl)
              n64 = Add(x=w322, y=w323) -> (x+y=w307:dbl)
              "Voltage" <- w307
              n65 = property on="Ei" class="Ref (strict)"() -> ("Value"=w282:refnum<k24>)  [unwired: 2 in, 2 out]
              n66 = property class="EI"(reference=w282, error in=w306, "Bandwidth"="Bandwidth 2", "CellOnOff"=w308, "CurrentRange"=w305, "Mode"=w303, "Setpoint"=w307) -> (error out=w287:errorcluster)  [unwired: 1 out]
              n67 = Equal To 0?(x=w320) -> (x = 0?=w321:bool)
              n68 = case shown="False" w321 {
                tunnel: w287 -> [w332 w335]
                tunnel: [w332 w335] -> w299
                frame False {
                }
                frame True {
                  n69 = property on="Equilibration \ntime (s)" class="DigNum (strict)"() -> ("Value"=w333:u32)  [unwired: 2 in, 2 out]
                  n70 = Multiply(x=u32 1000, y=w333) -> (x*y=w334:u32)
                  n71 = Wait (ms)(milliseconds to wait=w334) -> ()  [unwired: 1 out]
                }
              }
              n72 = property on="Sampler 2" class="Ref (strict)"() -> ("Value"=w280:refnum<k24>)  [unwired: 2 in, 2 out]
              n73 = property class="EI"(reference=w282, error in=w287) -> (error out=w286:errorcluster, "EiStatusSupportedFor"=→"EI status supported for":string[])  [unwired: 1 out]
              n74 = invoke class="Sampler" method="Sample"(reference=w280, error in=w287) -> (error out=w285:errorcluster)  [unwired: 1 in, 2 out]
              n75 = Build Array (concatenate)(w307, w319) -> (w318:dbl[])
              n76 = property class="EI"(reference=w282, error in=w299) -> (reference out=w281:refnum<k24>, error out=w298:errorcluster, "Bandwidth"=→"Bandwidth":i32, "CurrentRange"=→"CurrentRange":i32, "Mode"=→"Mode":i32, "Setpoint"=w296:dbl, "Current"=w297:dbl)
              "Measured voltage" <- w296
              n77 = flat-sequence {
                tunnel: w298 -> [w330]
                tunnel: [w330] -> w284
                tunnel: [w329] -> w304
                tunnel: w297 -> [w328]
                tunnel: w296 -> [w327]
                frame #0 {
                  n78 = Wait (ms)(milliseconds to wait=u32 100) -> ()  [unwired: 1 out]
                  n79 = call "Range_selector.vi"("potential"=w327, "current"=w328) -> ("range integer"=w329:i32)  [unwired: 9 in]
                }
              }
              n80 = Merge Errors(w284, w286, w285) -> (w283:errorcluster)
              n81 = call "P_Stat_Status1.vi"("error in (no error)"=w283, ".NET Refnum in"=w281) -> ("error out"=w289:errorcluster, "ManualCellSwitch"=→"ManualCellSwitch":bool, "Oscillation"=→"Oscillation":bool, "TemperatureOverload"=→"TemperatureOverload":bool, "CurrentOverload"=→"CurrentOverload":bool, "Cell"=→"Cell on?":bool)  [unwired: 3 in, 1 out]
              n82 = property class="EI"(reference=w281, error in=w289) -> (error out=w295:errorcluster, "Current"=w279:dbl)  [unwired: 1 out]
              "current" <- w279
              n83 = Bundle By Name(cluster=w315, "Current"=w279) -> (w314:T11)
              n84 = property on="current" class="DigNum (strict)"("Value"=w279) -> ()  [unwired: 2 in, 2 out]
              n85 = Build Array (concatenate)(w279, w317) -> (w316:dbl[])
            }
            frame "Wait" {
              n86 = Multiply(x="Wait before \nspectrum (s)", y=1000.0) -> (x*y=w345:dbl)
              n87 = Wait (ms)(milliseconds to wait=w345) -> ()  [unwired: 1 out]
              n88 = case shown="False" "Use iDus?" {
                tunnel: [SECenumctl."Read spectrum from Ocean" SECenumctl."Read spectrum from iDus"] -> w351
                frame False {
                }
                frame True {
                }
              }
              n89 = case shown="False" w340 {
                selector: w340 -> [w354 w357]
                tunnel: [0.0 1.0] -> w349
                tunnel: [1.0 ("Stop \npotential") 0.0 ("Stop \npotential")] -> w348
                tunnel: [w354 w357] -> w339
                frame False {
                }
                frame True {
                }
              }
            }
            frame "Read spectrum from iDus" {
              n90 = Unbundle By Name(w365) -> ("Exposure time"=w373:i32, "Number of scans in kinetic cycle"=w366:i32)
              n91 = Equal?(x=w372, y=2) -> (x = y?=w370:bool)
              n92 = Multiply(x=1024, y=w366) -> (x*y=w383:i32)
              n93 = stacked-sequence {
                seq-local: [_ _ _ _ _ _ _ _ _ _ w416 _] -> [_ _ _ _ _ _ _ _ _ _ _ w425]
                tunnel: [_ _ _ _ _ _ _ _ _ _ _ w426] -> w381
                tunnel: w366 -> [_ _ _ _ _ w405 _ _ _ _ _ w424]
                tunnel: w383 -> [_ _ _ _ _ _ _ _ _ _ w417 _]
                tunnel: w373 -> [_ _ _ w401 _ _ _ _ _ _ _ _]
                frame #0 {
                  w398 = u16 3  # AcquisitionMode
                  n94 = call "SetAcquisitionMode.vi"("mode"=w398) -> ()  [unwired: 1 in, 2 out]
                }
                frame #1 {
                  w399 = u16 0  # ReadMode
                  n95 = call "SetReadMode.vi"("mode"=w399) -> ()  [unwired: 1 in, 2 out]
                }
                frame #2 {
                  n96 = call "SetTriggerMode.vi"("mode"=TriggerMode_mode_typedef."Internal") -> ()  [unwired: 1 in, 2 out]
                }
                frame #3 {
                  n97 = call "SetExposureTime.vi"("time"=w401) -> ()  [unwired: 1 in, 2 out]
                }
                frame #4 {
                  n98 = call "GetNumberVSSpeeds.vi"() -> ("number"=w404:i32)  [unwired: 3 in, 2 out]
                  n99 = Subtract(x=w404, y=1) -> (x-y=w402:i32)
                  n100 = call "SetVSSpeed.vi"("index"=w402) -> ()  [unwired: 1 in, 2 out]
                }
                frame #5 {
                  n101 = call "SetNumberKinetics.vi"("number"=w405) -> ()  [unwired: 1 in, 2 out]
                }
                frame #6 {
                  w409 = 0  # Auto Shutter
                  n102 = call "SetShutter.vi"("type"=Shutter_type_typedef."TTL High", "mode"=w409, "closingtime"=0, "openingtime"=0) -> ()  [unwired: 10 in, 2 out]
                }
                frame #7 {
                  n103 = call "GetAcquisitionTimings.vi"() -> ("exposure"=w410:sgl)  [unwired: 11 in, 4 out]
                  n104 = property on="Calculated exposure time" class="DigNum (strict)"("Value"=w410) -> ()  [unwired: 2 in, 2 out]
                }
                frame #8 {
                  n105 = call "StartAcquisition.vi"() -> ("DLL error code"=w411:u32)  [unwired: 2 in, 1 out]
                  n106 = property on="Start Aquisition return code" class="DigNum (strict)"("Value"=w411) -> ()  [unwired: 2 in, 2 out]
                }
                frame #9 {
                  n107 = while {
                    stop <- w414 continue-if-true
                    w415 = u16 72  # DRV ACQUIRING
                    n108 = call "GetStatus.vi"() -> ("DLL error code"=→"Get status return code":u32, "status"=w413:T18)  [unwired: 3 in, 1 out]
                    n109 = Equal?(x=w413, y=w415) -> (x = y?=w414:bool)
                  }
                }
                frame #10 {
                  n110 = flat-sequence {
                    tunnel: [w419] -> w418
                    tunnel: w417 -> [w419]
                    tunnel: [w423] -> w416
                    tunnel: w418 -> [w421]
                    frame #0 {
                    }
                    frame #1 {
                      n111 = call "GetAcquiredData.vi"("size"=w421) -> ("DLL error code"=w420:u32, "array"=w423:i32[])  [unwired: 2 in, 1 out]
                      n112 = Equal?(x=20002 ("DRV_SUCCESS"), y=w420) -> ()  [unwired: 1 out]
                      n113 = property on="get aquired data return code" class="DigNum (strict)"("Value"=w420) -> ()  [unwired: 2 in, 2 out]
                    }
                  }
                }
                frame #11 {
                  n114 = for {
                    N: w424 -> [_]
                    shift-right: [w428] -> w426
                    shift-left: i32[][] [] -> [w430]
                    tunnel: w425 -> [w429]
                    i -> [w433]
                    w431 = 1024 ("x")
                    n115 = Multiply(x=w431, y=w433) -> (x*y=w435:i32)
                    n116 = Equal To 0?(x=w433) -> (x = 0?=w434:bool)
                    n117 = Array Subset(array=w429, index=w435, length=w431) -> (w432:i32[])
                    n118 = case shown="False" w434 {
                      tunnel: w432 -> [w437 w440]
                      tunnel: w430 -> [w438 _]
                      tunnel: [w436 w439] -> w428
                      frame False {
                        n119 = Build Array (concatenate)(w438, w437) -> (w436:i32[][])
                      }
                      frame True {
                        n120 = Build Array(w440) -> (w439:i32[][])
                      }
                    }
                  }
                }
              }
              n121 = property on="Use autolab?" class="Bool (strict)"() -> ("Value"=w361:bool)  [unwired: 2 in, 2 out]
              n122 = case shown="True" w361 {
                tunnel: [SECenumctl."Apply potential" SECenumctl."Apply potential Autolab"] -> w360
                frame False {
                }
                frame True {
                }
              }
              n123 = Unbundle By Name(w365) -> ("Number of scans in kinetic cycle"=w367:i32)
              n124 = flat-sequence {
                tunnel: [w446] -> w363
                tunnel: w381 -> [w444]
                tunnel: w367 -> [w443]
                tunnel: [w441] -> w364
                frame #0 {
                  n125 = for {
                    N: 1023 -> [_]
                    tunnel: w444 -> [w451]
                    tunnel: [w452] -> w446 mode=indexing
                    tunnel: w443 -> [w449]
                    tunnel: [w447] -> w441 mode=indexing
                    i -> [w448]
                    n126 = Index Array(array=w451, index (col)=w448) -> (element=w450:i32[])  [unwired: 1 in]
                    n127 = Add Array Elements(numeric array=w450) -> (sum=w453:i32)
                    n128 = Increment(x=w448) -> (x+1=w447:i32)
                    n129 = Divide(x=w453, y=w449) -> (x/y=w452:dbl)
                  }
                  n130 = Bundle(w441, w446) -> (→"?":cluster{i32[], dbl[]})  [unwired: 1 in]
                }
              }
              n131 = case shown="True" w370 {
                tunnel: w369 -> [w388 _]
                tunnel: w363 -> [w387 w390]
                tunnel: [w386 w391] -> w368
                tunnel: w364 -> [_ w389]
                frame False {
                  n132 = Build Array (concatenate)(w388, w387) -> (w386:dbl[][])
                }
                frame True {
                  n133 = Build Array(w389, w390) -> (w391:dbl[][])
                }
              }
              n134 = case shown="False" w376 {
                selector: w376 -> [w392 w395]
                tunnel: [0.0 1.0] -> w378
                tunnel: [1.0 ("Stop \npotential") 0.0 ("Stop \npotential")] -> w377
                tunnel: [w392 w395] -> w375
                frame False {
                }
                frame True {
                }
              }
            }
            frame "Read spectrum from Ocean" {
              # "Building an matric of WL + intensities of multiple expts"
              n135 = Equal?(x=w468, y=2) -> (x = y?=w466:bool)
              n136 = Unbundle By Name(w459) -> ("Integration time"=w458:i32, "Continous strobe delay"=w457:i32)
              n137 = call "ReadSpectrum(SubVI).vi"("Continuous \nStrobe Delay"=w457, "Enter the \nInetegration Time"=w458) -> ("Spectrum Values"=w464:dbl[], "WL Values"=w465:dbl[], "Number of Spectrometers"=→"Number of Spectrometers":i32)  [unwired: 7 in]
              n138 = case shown="False" w466 {
                tunnel: w465 -> [_ w486]
                tunnel: w464 -> [w482 w485]
                tunnel: [w481 w484] -> w462
                tunnel: w461 -> [w483 _]
                frame False {
                  # "Matrix + int on i >3"
                  n139 = Build Array (concatenate)(w483, w482) -> (w481:dbl[][])
                }
                frame True {
                  # "WL + Int on =3"
                  n140 = Build Array(w486, w485) -> (w484:dbl[][])
                }
              }
              n141 = Bundle("WL Values"=w465, "Spectrum Values"=w464) -> (→"?":T5)  [unwired: 1 in]
              n142 = property on="Use autolab?" class="Bool (strict)"() -> ("Value"=w454:bool)  [unwired: 2 in, 2 out]
              n143 = case shown="False" w454 {
                tunnel: [SECenumctl."Apply potential" SECenumctl."Apply potential Autolab"] -> w455
                frame False {
                }
                frame True {
                }
              }
              n144 = case shown="False" w460 {
                tunnel: [0.0 1.0] -> w474
                tunnel: [1.0 ("Stop \npotential") 0.0 ("Stop \npotential")] -> w473
                frame False {
                }
                frame True {
                }
              }
            }
          }
          n145 = case shown="False" w209 {
            tunnel: w221 -> [w231 w233]
            tunnel: w219 -> [w230 w232]
            tunnel: [w229 w234] -> w208
            frame False {
              n146 = Greater Or Equal?(x=w231, y=w230) -> (x >= y?=w229:bool)
            }
            frame True {
              n147 = Less Or Equal?(x=w233, y=w232) -> (x <= y?=w234:bool)
            }
          }
        }
        n148 = Unbundle By Name(w157) -> ("Default\n potential"=w179:dbl)
        n149 = property on="Use autolab?" class="Bool (strict)"() -> ("Value"=w152:bool)  [unwired: 2 in, 2 out]
        n150 = Insert Into Array(array=w159, index=0, new element=0.0 ("new element/subarray")) -> (w169:dbl[])
        n151 = Transpose Matrix(1:w173) -> (0:w172:dbl[][])
        n152 = Bundle(w159, w163) -> (→"?":cluster{dbl[], dbl[]})  [unwired: 1 in]
        n153 = Reverse 1D Array(array=w169) -> (reversed array=w168:dbl[])
        n154 = property on="V (during measurment)" class="DigNum (strict)"("Value"=w179) -> ()  [unwired: 2 in, 2 out]
        n155 = case shown="True" w152 {
          tunnel: w179 -> [w187 w189]
          frame False {
            n156 = call "IV setpotential.vi"("value"=w187) -> ()  [unwired: 8 in, 3 out]
          }
          frame True {
            n157 = property on="Ei" class="Ref (strict)"() -> ("Value"=w188:refnum<k24>)  [unwired: 2 in, 2 out]
            n158 = property class="EI"(reference=w188, "Setpoint"=w189) -> ()  [unwired: 1 in, 2 out]
          }
        }
        n159 = Replace Array Subset(array=w172, new element=w168, index (row)=0 ("index")) -> (w156:dbl[][])  [unwired: 1 in]
        n160 = Bundle By Name(cluster=w157, "Spectrum"=w172, "Current array"=w163, "Potential array"=w159) -> (w158:T11)
        n161 = Build Array(w159, w163) -> (w171:dbl[][])
        n162 = disable-structure shown="Enabled" {
          disable-tunnel: w156 -> [w205 _]
          disable-tunnel: w157 -> [w204 _]
          frame Enabled {
            n163 = call "WriteSEC.vi"("Init cluster"=w204, "Array"=w205) -> ()  [unwired: 10 in]
          }
          frame Disabled {
          }
        }
        n164 = Transpose Matrix(1:w171) -> (0:w170:dbl[][])
        n165 = disable-structure shown="Enabled" {
          disable-tunnel: w170 -> [w203 _]
          disable-tunnel: w158 -> [w202 _]
          frame Enabled {
            n166 = call "Write_JV.vi"("Init cluster"=w202, "Array"=w203) -> ()  [unwired: 10 in]
          }
          frame Disabled {
          }
        }
      }
      frame "Exit" {
        w487 = TRUE  # Stop Loop?
        w490 = State."Exit"  # (Value Not Used)
        # "Switch cell on/off"
        # "Diconnect device and close Ivium remdriver"
        # "Disconnect Ivium device (when connected)\nbefore terminating this VI"
        # "Exit - Exit the application."
        n167 = property on="Use autolab?" class="Bool (strict)"() -> ("Value"=w488:bool)  [unwired: 2 in, 2 out]
        n168 = case shown="True" w488 {
          tunnel: [w502 w520] -> w494
          tunnel: w493 -> [w499 w515]
          tunnel: [w497 0 ("devconnect")] -> w492
          frame False {
            w495 = FALSE ("Shut down sequence run?")
            # "This re-initialises a display for the iDus camera"
            # "On"
            # "Close Ivium Driver"
            n169 = To Long Integer(number=0) -> (32bit integer=w501:i32)
            n170 = call "IV setcellon.vi"("error in (no error)"=w499, "cellon"=w501) -> ("error out"=w498:errorcluster)  [unwired: 7 in, 2 out]
            n171 = call "IV getdevicestatus.vi"("error in (no error)"=w498) -> ("error out"=w503:errorcluster, "return type"=w504:i32)  [unwired: 9 in]
            n172 = Greater Than 0?(x=w504) -> (x > 0?=w496:bool)
            n173 = case shown="False" w496 {
              tunnel: [w507 w509] -> w505
              tunnel: w503 -> [w507 _]
              tunnel: [0 ("devconnect") w508] -> w497
              frame False {
              }
              frame True {
                w508 = 0 ("devconnect")
                n174 = call "IV connect.vi"("devconnect"=w508) -> ("error out"=w509:errorcluster)  [unwired: 8 in, 2 out]
              }
            }
            n175 = property on="Shut down sequence run?" class="Bool (strict)"("Value"=w495) -> ()  [unwired: 2 in, 2 out]
            n176 = property on="Return detector \nto room T?" class="Bool (strict)"("Value"=w495) -> ()  [unwired: 2 in, 2 out]
            n177 = call "IV close.vi"("error in (no error)"=w505) -> ("error out"=w502:errorcluster)  [unwired: 9 in, 1 out]
          }
          frame True {
            w514 = 0 items=["Off", "On"] ("CellOnOff")
            n178 = property on="Ei" class="Ref (strict)"() -> ("Value"=w513:refnum<k24>)  [unwired: 2 in, 2 out]
            n179 = property class="EI"(reference=w513, error in=w515, "CellOnOff"=w514) -> (error out=w512:errorcluster)  [unwired: 1 out]
            n180 = property on="ManualCellSwitch" class="Bool (strict)"("Value"=FALSE ("ManualCellSwitch")) -> ()  [unwired: 2 in, 2 out]
            n181 = property on="Cell on?" class="Bool (strict)"("Value"=FALSE ("Cell")) -> ()  [unwired: 2 in, 2 out]
            n182 = property on="instrument" class="Ref (strict)"(error in=w512) -> (error out=w518:errorcluster, "Value"=w519:refnum<k24>)  [unwired: 1 in, 1 out]
            n183 = property on="Autolab Connected?" class="Bool (strict)"("Value"=FALSE ("IsConnected")) -> ()  [unwired: 2 in, 2 out]
            n184 = invoke class="Instrument" method="Disconnect"(reference=w519, error in=w518) -> (error out=w520:errorcluster)  [unwired: 1 in, 2 out]
          }
        }
        n185 = property on="V2 applied?" class="Bool (strict)"("Value"=FALSE ("V2 applied")) -> ()  [unwired: 2 in, 2 out]
      }
      frame "Run OSPEC" {
        n186 = property on="Use autolab?" class="Bool (strict)"() -> ("Value"=w521:bool)  [unwired: 2 in, 2 out]
        n187 = case shown="True" w521 {
          tunnel: w528 -> [w532 w540]
          tunnel: [w531 w540] -> w527
          frame False {
            # "Get cell status"
            # "Get Device Status"
            # "Direct Mode"
            n188 = call "IV getdevicestatus.vi"() -> ("return type"=w535:i32)  [unwired: 10 in, 1 out]
            n189 = Increment(x=w535) -> (x+1=w534:i32)
            n190 = case shown="0, Default" w534 {
              tunnel: ["no IviumSoft" "device not connected" "device available_idle" "device available_busy"] -> w533
              frame 0, Default {
              }
              frame 1 {
              }
              frame 2 {
              }
              frame 3 {
              }
            }
            n191 = Bundle By Name(cluster=w532, "Status"=w533) -> (w531:T11)
          }
          frame True {
          }
        }
        n192 = while {
          shift-right: [w541] -> w525
          shift-left: w526 -> [w546]
          shift-right: [w542] -> w524
          shift-left: w527 -> [w548]
          shift-right: [w545] -> _
          shift-left: OSSPEC."Apply V1" -> [w547]
          i -> [w544]
          stop <- w543 stop-if-true
          n193 = case shown="\"Read Potential and spectrum\", Default" w547 {
            tunnel: w548 -> [w552 w880 w1374 w1396 w1458 w1524]
            tunnel: w546 -> [w551 w897 w1378 w1395 w1468 w1549]
            tunnel: [OSSPEC."End measurment" w913 OSSPEC."Read Potential and spectrum" OSSPEC."Read current and spectrum" OSSPEC."Read current and spectrum" OSSPEC."End measurment"] -> w545
            tunnel: [w557 w896 w1377 w1391 w1459 w1546] -> w541
            tunnel: [w558 w904 w1374 w1392 w1458 w1524] -> w542
            tunnel: w544 -> [_ _ _ _ _ _]
            tunnel: [FALSE FALSE FALSE FALSE FALSE TRUE] -> w543
            frame "Read Potential and spectrum", Default {
              n194 = property on="Use autolab?" class="Bool (strict)"() -> ("Value"=w549:bool)  [unwired: 2 in, 2 out]
              n195 = case shown="True" w549 {
                tunnel: w551 -> [w572 w584]
                tunnel: [w571 w582] -> w550
                frame False {
                  n196 = flat-sequence {
                    tunnel: w572 -> [w575]
                    tunnel: [w575] -> w573
                    tunnel: [w576] -> w571
                    tunnel: w573 -> [w577]
                    frame #0 {
                      n197 = Wait (ms)(milliseconds to wait=u32 50) -> ()  [unwired: 1 out]
                    }
                    frame #1 {
                      n198 = To Long Integer(number=T17."IStat4EL" ("Configuration")) -> (32bit integer=w579:i32)
                      n199 = call "IV setconnectionmode.vi"("error in (no error)"=w577, "value"=w579) -> ("error out"=w576:errorcluster)  [unwired: 7 in, 2 out]
                    }
                  }
                }
                frame True {
                  w580 = 1 items=["Off", "On"] ("CellOnOff")
                  w585 = -4 items=["CR07_1A"=0, "CR06_10A"=1, "CR01_100A"=2, "CR00_1000A"=3, "CR05_20A"=20, "CR04_40A"=40, "CR03_50A"=60, "CR02_80A"=80, "CR19_1pA"=-12, "CR18_10pA"=-11, "CR17_100pA"=-10, "CR16_1nA"=-9, "CR15_10nA"=-8, "CR14_100nA"=-7, "CR13_1uA"=-6, "CR12_10uA"=-5, "CR11_100uA"=-4, "CR10_1mA"=-3, "CR09_10mA"=-2, "CR08_100mA"=-1] ("CurrentRange")
                  w587 = 1 items=["Potentiostatic", "Galvanostatic"] ("Mode")
                  n200 = property on="Ei" class="Ref (strict)"() -> ("Value"=w581:refnum<k24>)  [unwired: 2 in, 2 out]
                  n201 = property class="EI"(reference=w581, error in=w584, "CurrentRange"=w585) -> (error out=w583:errorcluster)  [unwired: 1 out]
                  n202 = property class="EI"(reference=w581, error in=w583, "Mode"=w587, "Setpoint"=0.0, "CellOnOff"=w580) -> (error out=w582:errorcluster)  [unwired: 1 out]
                }
              }
              n203 = Unbundle By Name(w552) -> ("Spectrum"=w560:dbl[][])
              n204 = Unbundle By Name(w552) -> ("Time for spectrum measurment"=w559:i32[], "Start time"=w562:i32)
              n205 = Unbundle By Name(w552) -> ("Potential array"=w555:dbl[])
              n206 = property on="Use iDus?" class="Bool (strict)"() -> ("Value"=w553:bool)  [unwired: 2 in, 2 out]
              n207 = Unbundle By Name(w552) -> ("Time for E measurment"=w554:i32[], "Start time"=w561:i32)
              n208 = while {
                shift-right: [w800] -> _
                shift-left: w552 -> [w801]
                shift-right: [w792] -> _
                shift-left: OSPEC-enum."Wait" -> [w802]
                shift-right: [w799] -> w565
                shift-left: w554 -> [w798]
                shift-right: [w793] -> w564
                shift-left: w555 -> [w796]
                shift-right: [w795] -> _
                shift-left: w561 -> [w794]
                shift-right: [w790] -> w557
                shift-left: w550 -> [w791]
                i -> [w797]
                stop <- w787 stop-if-true
                n209 = case shown="\"Read\", Default" w802 {
                  tunnel: w801 -> [w808 w819 w875]
                  tunnel: [w808 w819 w875] -> w800
                  tunnel: [w806 FALSE FALSE] -> w789
                  tunnel: [w812 w823 w873] -> w799
                  tunnel: w798 -> [w812 w824 w873]
                  tunnel: w797 -> [_ w828 _]
                  tunnel: [w810 w827 w870] -> w793
                  tunnel: w796 -> [w810 w826 w870]
                  tunnel: [w807 w820 w872] -> w795
                  tunnel: w794 -> [w807 _ w872]
                  tunnel: [OSPEC-enum."Wait" OSPEC-enum."Check exit" OSPEC-enum."Read"] -> w792
                  tunnel: w791 -> [w809 w816 w869]
                  tunnel: [w809 w815 w869] -> w790
                  frame "Check exit" {
                    n210 = Unbundle By Name(w808) -> ("V off time"=w804:dbl)
                    n211 = Multiply(x=w804, y=1000.0) -> (x*y=w805:dbl)
                    n212 = Greater Or Equal?(x=w807, y=w805) -> (x >= y?=w806:bool)
                  }
                  frame "Read", Default {
                    # "Building a 1d matrix of potentials and times"
                    n213 = property on="Use autolab?" class="Bool (strict)"() -> ("Value"=w813:bool)  [unwired: 2 in, 2 out]
                    n214 = case shown="True" w813 {
                      tunnel: [w831 w834] -> w817
                      tunnel: w816 -> [w830 w832]
                      tunnel: [w829 w833] -> w815
                      frame False {
                        n215 = call "IV getpotential.vi"("error in (no error)"=w830) -> ("error out"=w829:errorcluster, "value out"=w831:dbl)  [unwired: 8 in, 1 out]
                      }
                      frame True {
                        n216 = disable-structure shown="Disabled" {
                          disable-tunnel: [w839 w849] -> w834
                          disable-tunnel: [w838 w851] -> w833
                          disable-tunnel: w832 -> [w836 w859]
                          frame Enabled {
                            n217 = property on="Ei" class="Ref (strict)"() -> ("Value"=w837:refnum<k24>)  [unwired: 2 in, 2 out]
                            n218 = disable-structure shown="Disabled" {
                              disable-tunnel: w837 -> [w847 _]
                              disable-tunnel: w836 -> [w843 w848]
                              disable-tunnel: [w842 w848] -> w835
                              frame Disabled {
                                w844 = -4 items=["CR07_1A"=0, "CR06_10A"=1, "CR01_100A"=2, "CR00_1000A"=3, "CR05_20A"=20, "CR04_40A"=40, "CR03_50A"=60, "CR02_80A"=80, "CR19_1pA"=-12, "CR18_10pA"=-11, "CR17_100pA"=-10, "CR16_1nA"=-9, "CR15_10nA"=-8, "CR14_100nA"=-7, "CR13_1uA"=-6, "CR12_10uA"=-5, "CR11_100uA"=-4, "CR10_1mA"=-3, "CR09_10mA"=-2, "CR08_100mA"=-1] ("CurrentRange")
                                w846 = 1 items=["Potentiostatic", "Galvanostatic"] ("Mode")
                                n219 = property class="EI"(reference=w847, error in=w843, "Mode"=w846, "Setpoint"=0.0, "CurrentRange"=w844) -> (error out=w842:errorcluster)  [unwired: 1 out]
                              }
                              frame Enabled {
                              }
                            }
                            n220 = property class="EI"(reference=w837, error in=w835) -> (error out=w838:errorcluster, "Current"=w840:dbl, "Potential"=w839:dbl)  [unwired: 1 out]
                            n221 = disable-structure shown="Disabled" {
                              disable-tunnel: w840 -> [w841 _]
                              frame Disabled {
                                "OCP I (close to 0)" <- w841
                              }
                              frame Enabled {
                              }
                            }
                          }
                          frame Disabled {
                            w856 = -4 items=["CR07_1A"=0, "CR06_10A"=1, "CR01_100A"=2, "CR00_1000A"=3, "CR05_20A"=20, "CR04_40A"=40, "CR03_50A"=60, "CR02_80A"=80, "CR19_1pA"=-12, "CR18_10pA"=-11, "CR17_100pA"=-10, "CR16_1nA"=-9, "CR15_10nA"=-8, "CR14_100nA"=-7, "CR13_1uA"=-6, "CR12_10uA"=-5, "CR11_100uA"=-4, "CR10_1mA"=-3, "CR09_10mA"=-2, "CR08_100mA"=-1] ("CurrentRange")
                            w860 = 0 items=["Off", "On"] ("CellOnOff")
                            w861 = 2 items=["UltraHigh_Speed", "High_Speed", "High_Stability"] ("Bandwidth")
                            w862 = 0 items=["Potentiostatic", "Galvanostatic"] ("Mode")
                            w866 = 0 items=["Potentiostatic", "Galvanostatic"] ("Mode")
                            w867 = 0 items=["Off", "On"] ("CellOnOff")
                            w868 = 2 items=["UltraHigh_Speed", "High_Speed", "High_Stability"] ("Bandwidth")
                            n222 = property on="Ei" class="Ref (strict)"() -> ("Value"=w858:refnum<k24>)  [unwired: 2 in, 2 out]
                            n223 = property on="Sampler 2" class="Ref (strict)"() -> ("Value"=w857:refnum<k24>)  [unwired: 2 in, 2 out]
                            n224 = call "EI (A).vi"("Sampler"=w857, "Ei"=w858, "CellOnOff"=w867, "Bandwidth"=w868, "CurrentRange"=w856, "Mode"=w866, "error in (no error)"=w859, "Disable Sampler"=FALSE) -> ("Cell"=w855:bool, "PotentialOverload"=w854:bool, "error out"=w852:errorcluster)  [unwired: 6 in, 11 out]
                            n225 = property on="PotentialOverload" class="Bool (strict)"("Value"=w854) -> ()  [unwired: 2 in, 2 out]
                            n226 = property on="Cell on?" class="Bool (strict)"("Value"=w855) -> ()  [unwired: 2 in, 2 out]
                            n227 = call "Sampler.vi"("error in (no error)"=w859, "Sampler"=w857) -> ("error out"=w864:errorcluster)  [unwired: 7 in, 2 out]
                            n228 = Merge Errors(w864, w852) -> (w865:errorcluster)
                            n229 = call "EI (A).vi"("Sampler"=w857, "Ei"=w858, "CellOnOff"=w860, "Bandwidth"=w861, "Mode"=w862, "error in (no error)"=w865, "Disable Sampler"=FALSE) -> ("Potential"=w849:dbl, "Current"=w850:dbl, "error out"=w851:errorcluster)  [unwired: 7 in, 11 out]
                            n230 = property on="current" class="DigNum (strict)"("Value"=w850) -> ()  [unwired: 2 in, 2 out]
                            n231 = property on="Voltage" class="DigNum (strict)"("Value"=w849) -> ()  [unwired: 2 in, 2 out]
                          }
                        }
                      }
                    }
                    "OCP" <- w817
                    n232 = Unbundle By Name(w819) -> ("Start time"=w818:i32)
                    n233 = Tick Count (ms)() -> (millisecond timer value=w814:u32)
                    n234 = Subtract(x=w814, y=w818) -> (x-y=w820:u32)
                    n235 = Equal?(x=1, y=w828) -> ()  [unwired: 1 out]
                    n236 = Build Array (concatenate)(w826, w817) -> (w827:dbl[])
                    n237 = Build Array (concatenate)(w824, w820) -> (w823:u32[])
                  }
                  frame "Wait" {
                    n238 = Unbundle By Name(w875) -> ("Sample rate"=w876:dbl)
                    n239 = Multiply(x=w876, y=1000.0) -> (x*y=w878:dbl)
                    n240 = Wait (ms)(milliseconds to wait=w878) -> ()  [unwired: 1 out]
                  }
                }
                n241 = property on="IDus not in read loop? (kinetic)" class="Bool (strict)"() -> ("Value"=w788:bool)  [unwired: 2 in, 2 out]
                n242 = And(x=w788, y=w789) -> (x .and. y?=w787:bool)
              }
              n243 = case shown="True" w553 {
                tunnel: [w599 w662] -> w567
                tunnel: [w598 w663] -> w566
                tunnel: w562 -> [w597 w669]
                tunnel: w560 -> [w596 w667]
                tunnel: w559 -> [w594 w665]
                tunnel: [w593 w664] -> w556
                tunnel: w552 -> [w592 w668]
                frame False {
                  n244 = local read "Wrapper Out"() -> (w590:u32)
                  n245 = local read "ContinuousStrobe Out"() -> (w591:u32)
                  n246 = local read "WL Values"() -> (w589:dbl[])
                  n247 = while {
                    shift-right: [w615] -> _
                    shift-left: w592 -> [w616]
                    shift-right: [w608] -> _
                    shift-left: OSPEC-enum."Read" -> [w617]
                    shift-right: [w613] -> w598
                    shift-left: w594 -> [w612]
                    shift-right: [w607] -> w593
                    shift-left: w596 -> [w611]
                    shift-right: [w610] -> w599
                    shift-left: w597 -> [w601]
                    tunnel: w590 -> [w606]
                    tunnel: [w605] -> w595
                    tunnel: w591 -> [w604]
                    tunnel: w589 -> [w603]
                    tunnel: [w602] -> w588
                    i -> [w609]
                    stop <- w614 stop-if-true
                    n248 = case shown="\"Check exit\"" w617 {
                      tunnel: w616 -> [w626 w632 w656]
                      tunnel: [w626 w632 w656] -> w615
                      tunnel: [w624 FALSE FALSE] -> w614
                      tunnel: [w628 w644 w654] -> w613
                      tunnel: w612 -> [w628 w643 w654]
                      tunnel: w609 -> [_ _ _]
                      tunnel: [w623 w638 w650] -> w607
                      tunnel: w611 -> [w623 w642 w650]
                      tunnel: [w625 w629 w647] -> w610
                      tunnel: w601 -> [w625 _ w647]
                      tunnel: [OSPEC-enum."Wait" OSPEC-enum."Check exit" OSPEC-enum."Read"] -> w608
                      tunnel: w606 -> [w621 w636 w651]
                      tunnel: [w622 w637 w652] -> w605
                      tunnel: w604 -> [w622 w637 w652]
                      tunnel: w603 -> [_ w635 _]
                      tunnel: [w621 w636 w651] -> w602
                      frame "Check exit" {
                        n249 = Unbundle By Name(w626) -> ("V off time"=w620:dbl)
                        n250 = Multiply(x=w620, y=1000.0) -> (x*y=w618:dbl)
                        n251 = Greater Or Equal?(x=w625, y=w618) -> (x >= y?=w624:bool)
                      }
                      frame "Read", Default {
                        # "Continue 2d matrix of specta"
                        # "Continue to add times to this"
                        n252 = call "Wrapper_getSpectrum.vi"("Index"=0, "Wrapper"=w636) -> ("Spectrum Values"=w634:dbl[])  [unwired: 1 out]
                        n253 = Tick Count (ms)() -> (millisecond timer value=w630:u32)
                        n254 = Unbundle By Name(w632) -> ("Start time"=w631:i32)
                        n255 = Subtract(x=w630, y=w631) -> (x-y=w629:u32)
                        "Time during PD" <- w629
                        n256 = Bundle("WL Values"=w635, "Spectrum Values"=w634) -> (→"?":T5)  [unwired: 1 in]
                        n257 = Build Array (concatenate)(w643, w629) -> (w644:u32[])
                        n258 = Build Array (concatenate)(w642, w634) -> (w638:dbl[][])
                      }
                      frame "Wait" {
                        n259 = Unbundle By Name(w656) -> ("Sample rate"=w657:dbl)
                        n260 = Multiply(x=1000.0, y="Slow sample time (s)") -> (x*y=w646:dbl)
                        n261 = Greater?(x=w647, y=w646) -> (0:w645:bool)
                        n262 = case shown="True" w645 {
                          tunnel: w657 -> [w658 _]
                          frame False {
                            n263 = Multiply(x=w658, y=1000.0) -> (x*y=w660:dbl)
                            n264 = Wait (ms)(milliseconds to wait=w660) -> ()  [unwired: 1 out]
                          }
                          frame True {
                            # "slow down read to measure slow decays\nwithout oversampling"
                            n265 = Wait (ms)(milliseconds to wait=u32 500) -> ()  [unwired: 1 out]
                          }
                        }
                      }
                    }
                  }
                  n266 = call "End spectrum measurment.vi"("ContinuousStrobe Out"=w595, "Wrapper Out"=w588) -> ()  [unwired: 10 in]
                }
                frame True {
                  n267 = while {
                    shift-right: [w679] -> w662
                    shift-left: w669 -> [w680]
                    shift-right: [w672] -> _
                    shift-left: OSPEC-enum."Wait" -> [w681]
                    shift-right: [w678] -> w663
                    shift-left: w665 -> [w677]
                    shift-right: [w671] -> w664
                    shift-left: w667 -> [w676]
                    shift-right: [w675] -> _
                    shift-left: w668 -> [w674]
                    i -> [w673]
                    stop <- w670 stop-if-true
                    n268 = case shown="\"Wait\"" w681 {
                      tunnel: w680 -> [w683 _ w784]
                      tunnel: [w683 w692 w784] -> w679
                      tunnel: [w689 FALSE FALSE] -> w670
                      tunnel: [w691 w696 w782] -> w678
                      tunnel: w677 -> [w691 w700 w782]
                      tunnel: w673 -> [_ w703 _]
                      tunnel: w676 -> [w684 w699 w778]
                      tunnel: [w690 w694 w780] -> w675
                      tunnel: w674 -> [w690 w694 w780]
                      tunnel: [OSPEC-enum."Wait" OSPEC-enum."Check exit" OSPEC-enum."Read"] -> w672
                      tunnel: [w684 w697 w778] -> w671
                      frame "Check exit" {
                        n269 = Unbundle By Name(w690) -> ("V off time"=w685:dbl)
                        n270 = Multiply(x=w685, y=1000.0) -> (x*y=w686:dbl)
                        n271 = Greater Or Equal?(x=w683, y=w686) -> (x >= y?=w689:bool)
                      }
                      frame "Read", Default {
                        n272 = Unbundle By Name(w694) -> ("Start time"=w693:i32)
                        n273 = property on="Number of scans in kinetic cycle" class="DigNum (strict)"() -> ("Value"=w695:i32)  [unwired: 2 in, 2 out]
                        n274 = Tick Count (ms)() -> (millisecond timer value=w701:u32)
                        n275 = call "GetDetector.vi"() -> ("xpixels"=w702:i32)  [unwired: 4 in, 3 out]
                        n276 = Subtract(x=w701, y=w693) -> (x-y=w692:u32)
                        n277 = Equal?(x=w703, y=1.0) -> (x = y?=w698:bool)
                        n278 = stacked-sequence {
                          seq-local: [_ _ _ _ _ _ _ _ _ _ w737 _] -> [_ _ _ _ _ _ _ _ _ _ _ w757]
                          seq-local: [_ _ _ _ _ _ _ _ w722 _ _ _] -> [_ _ _ _ _ _ _ _ _ _ _ w755]
                          seq-local: [_ _ _ _ _ _ _ _ _ _ w736 _] -> [_ _ _ _ _ _ _ _ _ _ _ w756]
                          tunnel: [_ _ _ _ _ _ _ _ _ _ _ w750] -> w697
                          tunnel: [_ _ _ _ _ _ _ _ _ _ _ w751] -> w696
                          tunnel: w695 -> [_ _ _ _ _ w715 _ _ _ _ _ w749]
                          tunnel: w692 -> [_ _ _ _ _ _ _ _ _ _ _ w752]
                          tunnel: w692 -> [_ _ _ _ _ _ _ _ _ _ _ _]
                          tunnel: w702 -> [_ w708 _ _ _ _ _ _ _ _ _ _]
                          tunnel: w693 -> [_ _ _ _ _ _ _ _ w721 _ w735 _]
                          tunnel: w700 -> [_ _ _ _ _ _ _ _ _ _ _ w748]
                          tunnel: w699 -> [_ _ _ _ _ _ _ _ _ _ _ w747]
                          tunnel: w698 -> [_ _ _ _ _ _ _ _ _ _ _ w746]
                          frame #0 {
                            w707 = u16 3  # AcquisitionMode
                            n279 = call "SetAcquisitionMode.vi"("mode"=w707) -> ()  [unwired: 1 in, 2 out]
                          }
                          frame #1 {
                            w709 = u16 0  # ReadMode
                            n280 = property on="xpixels" class="DigNum (strict)"("Value"=w708) -> ()  [unwired: 2 in, 2 out]
                            n281 = call "SetReadMode.vi"("mode"=w709) -> ()  [unwired: 1 in, 2 out]
                          }
                          frame #2 {
                            n282 = call "SetTriggerMode.vi"("mode"=TriggerMode_mode_typedef."Internal") -> ()  [unwired: 1 in, 2 out]
                          }
                          frame #3 {
                            n283 = property on="Exposure time (s)" class="DigNum (strict)"() -> ("Value"=w711:dbl)  [unwired: 2 in, 2 out]
                            n284 = call "SetExposureTime.vi"("time"=w711) -> ()  [unwired: 1 in, 2 out]
                          }
                          frame #4 {
                            n285 = call "GetNumberVSSpeeds.vi"() -> ("number"=w714:i32)  [unwired: 3 in, 2 out]
                            n286 = Subtract(x=w714, y=1) -> (x-y=w712:i32)
                            n287 = call "SetVSSpeed.vi"("index"=w712) -> ()  [unwired: 1 in, 2 out]
                          }
                          frame #5 {
                            n288 = call "SetNumberKinetics.vi"("number"=w715) -> ()  [unwired: 1 in, 2 out]
                          }
                          frame #6 {
                            w718 = 0  # Auto Shutter
                            n289 = property on="Shutter open and close time" class="DigNum (strict)"() -> ("Value"=w716:i32)  [unwired: 2 in, 2 out]
                            n290 = property on="Shutter opens on TTL" class="Enum (strict)"() -> ("Value"=w717:T9)  [unwired: 2 in, 2 out]
                            n291 = call "SetShutter.vi"("type"=w717, "mode"=w718, "closingtime"=w716, "openingtime"=w716) -> ()  [unwired: 10 in, 2 out]
                          }
                          frame #7 {
                            # "Meybe delete the exposure time insupt here"
                            n292 = property on="Exposure time (s)" class="DigNum (strict)"() -> ("Value"=w720:dbl)  [unwired: 2 in, 2 out]
                            n293 = call "GetAcquisitionTimings.vi"("exposure input"=w720) -> ("exposure"=w719:sgl)  [unwired: 10 in, 4 out]
                            n294 = property on="Calculated exposure time" class="DigNum (strict)"("Value"=w719) -> ()  [unwired: 2 in, 2 out]
                          }
                          frame #8 {
                            n295 = flat-sequence {
                              tunnel: [w723] -> w722
                              tunnel: w721 -> [w724]
                              frame #0 {
                                n296 = Tick Count (ms)() -> (millisecond timer value=w725:u32)
                                n297 = Subtract(x=w725, y=w724) -> (x-y=w723:u32)
                                n298 = property on="Time before the start of current aquisition (ms)" class="DigNum (strict)"("Value"=w723) -> ()  [unwired: 2 in, 2 out]
                              }
                              frame #1 {
                                n299 = call "StartAcquisition.vi"() -> ("DLL error code"=w726:u32)  [unwired: 2 in, 1 out]
                                n300 = property on="Start Aquisition return code" class="DigNum (strict)"("Value"=w726) -> ()  [unwired: 2 in, 2 out]
                              }
                            }
                          }
                          frame #9 {
                            n301 = while {
                              stop <- w730 continue-if-true
                              w731 = u16 72  # DRV ACQUIRING
                              n302 = call "GetStatus.vi"() -> ("DLL error code"=w728:u32, "status"=w729:T18)  [unwired: 3 in, 1 out]
                              n303 = property on="Get status return code" class="DigNum (strict)"("Value"=w728) -> ()  [unwired: 2 in, 2 out]
                              n304 = Equal?(x=w729, y=w731) -> (x = y?=w730:bool)
                              n305 = property on="IDus not in read loop? (kinetic)" class="Bool (strict)"("Value"=FALSE ("IDus not in read loop? (kinetic)")) -> ()  [unwired: 2 in, 2 out]
                            }
                          }
                          frame #10 {
                            n306 = flat-sequence {
                              tunnel: [w738] -> w736
                              tunnel: w735 -> [w739]
                              tunnel: [w745] -> w737
                              tunnel: w734 -> [w742]
                              frame #0 {
                                n307 = Tick Count (ms)() -> (millisecond timer value=w740:u32)
                                n308 = Subtract(x=w740, y=w739) -> (x-y=w738:u32)
                                n309 = property on="Time  after the aquisition (before fetch data), (ms)" class="DigNum (strict)"("Value"=w738) -> ()  [unwired: 2 in, 2 out]
                              }
                              frame #1 {
                                n310 = call "GetAcquiredData.vi"("size"=w742) -> ("DLL error code"=w743:u32, "array"=w745:i32[])  [unwired: 2 in, 1 out]
                                n311 = Equal?(x=20002 ("DRV_SUCCESS"), y=w743) -> (x = y?=w741:bool)
                                n312 = property on="get aquired data return code" class="DigNum (strict)"("Value"=w743) -> ()  [unwired: 2 in, 2 out]
                                n313 = property on="Get aqisition ok? (kinetic mode)" class="Bool (strict)"("Value"=w741) -> ()  [unwired: 2 in, 2 out]
                              }
                            }
                            n314 = property on="Number of scans in kinetic cycle" class="DigNum (strict)"() -> ("Value"=w732:i32)  [unwired: 2 in, 2 out]
                            n315 = Multiply(x=1024.0, y=w732) -> (x*y=w734:dbl)
                          }
                          frame #11 {
                            n316 = Subtract(x=w756, y=w755) -> (x-y=w754:u32)
                            n317 = Divide(x=w754, y=w749) -> (x/y=w753:dbl)
                            n318 = for {
                              N: w749 -> [_]
                              tunnel: w757 -> [w771]
                              tunnel: w753 -> [w769]
                              tunnel: w752 -> [w767]
                              shift-right: [w765] -> w750
                              shift-left: w747 -> [w764]
                              shift-right: [w761] -> w751
                              shift-left: w748 -> [w762]
                              tunnel: w746 -> [_]
                              i -> [w759]
                              w766 = 1024 ("x")
                              n319 = Multiply(x=w759, y=w769) -> (x*y=w768:dbl)
                              n320 = Multiply(x=w766, y=w759) -> (x*y=w770:i32)
                              n321 = Add(x=w768, y=w767) -> (x+y=w763:dbl)
                              n322 = Array Subset(array=w771, index=w770, length=w766) -> (w758:i32[])
                              n323 = Equal To 0?(x=w759) -> (x = 0?=w760:bool)
                              n324 = case shown="True" w760 {
                                tunnel: w758 -> [_ w773]
                                frame False {
                                }
                                frame True {
                                n325 = for {
                                N: 1023 -> [_]
                                tunnel: [w776] -> w774 mode=indexing
                                i -> [w777]
                                n326 = Increment(x=w777) -> (x+1=w776:i32)
                                }
                                n327 = Bundle(w774, w773) -> (w772:cluster{i32[], i32[]})  [unwired: 1 in]
                                n328 = property class="XYGraph (strict)"("Value"=w772) -> ()  [unwired: 2 in, 2 out]
                                }
                              }
                              n329 = Build Array (concatenate)(w764, w758) -> (w765:dbl[][])
                              n330 = Build Array (concatenate)(w762, w763) -> (w761:dbl[])
                            }
                          }
                        }
                      }
                      frame "Wait" {
                        n331 = Unbundle By Name(w780) -> ("Sample rate"=w779:dbl)
                        n332 = Multiply(x=w779, y=1000.0) -> (x*y=w786:dbl)
                        n333 = Wait (ms)(milliseconds to wait=w786) -> ()  [unwired: 1 out]
                      }
                    }
                    n334 = case shown="True" w670 {
                      selector: w670 -> [_ w682]
                      frame False {
                      }
                      frame True {
                        n335 = property on="IDus not in read loop? (kinetic)" class="Bool (strict)"("Value"=w682) -> ()  [unwired: 2 in, 2 out]
                      }
                    }
                  }
                }
              }
              n336 = Bundle By Name(cluster=w552, "Time for spectrum measurment"=w566, "Time elapsed"=w567, "Spectrum"=w556) -> (w563:T11)
              n337 = Bundle By Name(cluster=w563, "Time for E measurment"=w565, "Potential array"=w564) -> (w558:T11)
            }
            frame "Read current and spectrum" {
              n338 = local read "V (during measurment)"() -> (w901:dbl)
              n339 = Unbundle By Name(w880) -> ("Time for spectrum measurment"=w895:i32[], "Start time"=w900:i32)
              n340 = Unbundle By Name(w880) -> ("V 1"=w902:dbl, "Spectrum"=w898:dbl[][])
              n341 = property on="squre wave" class="Bool (strict)"() -> ("Value"=w887:bool)  [unwired: 2 in, 2 out]
              n342 = property on="V2 applied?" class="Bool (strict)"() -> ("Value"=w886:bool)  [unwired: 2 in, 2 out]
              n343 = property on="Use iDus?" class="Bool (strict)"() -> ("Value"=w892:bool)  [unwired: 2 in, 2 out]
              n344 = Equal?(x=w901, y=w902) -> (x = y?=w884:bool)
              n345 = And(x=w887, y=w886) -> (x .and. y?=w882:bool)
              n346 = Not(x=w882) -> (.not. x?=w885:bool)
              n347 = And(x=w884, y=w885) -> (x .and. y?=w883:bool)
              n348 = Unbundle By Name(w880) -> ("Current array"=w894:dbl[])
              n349 = Unbundle By Name(w880) -> ("Time for I measurment"=w893:i32[], "Start time"=w899:i32)
              n350 = property on="V2 applied?" class="Bool (strict)"() -> ("Value"=w881:bool)  [unwired: 2 in, 2 out]
              n351 = case shown="False" w881 {
                tunnel: w880 -> [w916 w918]
                tunnel: [w915 w917] -> w879
                frame False {
                  n352 = Unbundle By Name(w916) -> ("V 1"=w915:dbl)
                }
                frame True {
                  n353 = Unbundle By Name(w918) -> ("V 2"=w917:dbl)
                }
              }
              n354 = while {
                shift-right: [w1209] -> _
                shift-left: w880 -> [w1210]
                shift-right: [w1201] -> _
                shift-left: OSPEC-enum."Wait" -> [w1211]
                shift-right: [w1208] -> w905
                shift-left: w893 -> [w1207]
                shift-right: [w1202] -> w891
                shift-left: w894 -> [w1205]
                shift-right: [w1204] -> _
                shift-left: w899 -> [w1203]
                tunnel: w883 -> [w1200]
                shift-right: [w1198] -> w896
                shift-left: w897 -> [w1199]
                tunnel: w879 -> [w1194]
                i -> [w1206]
                stop <- w1195 stop-if-true
                n355 = case shown="\"Read\", Default" w1211 {
                  tunnel: w1210 -> [w1223 w1254 w1360]
                  tunnel: [w1222 w1254 w1360] -> w1209
                  tunnel: [w1220 FALSE FALSE] -> w1196
                  tunnel: [w1225 w1262 w1358] -> w1208
                  tunnel: w1207 -> [w1225 w1263 w1358]
                  tunnel: w1206 -> [_ w1268 _]
                  tunnel: [w1217 w1267 w1355] -> w1202
                  tunnel: w1205 -> [w1217 w1266 w1355]
                  tunnel: [w1215 w1255 w1357] -> w1204
                  tunnel: w1203 -> [w1215 _ w1357]
                  tunnel: [OSPEC-enum."Wait" OSPEC-enum."Check exit" OSPEC-enum."Read"] -> w1201
                  tunnel: w1200 -> [_ w1257 _]
                  tunnel: w1199 -> [w1216 w1249 w1354]
                  tunnel: [w1216 w1252 w1354] -> w1198
                  tunnel: w1194 -> [_ w1248 _]
                  frame "Check exit" {
                    n356 = local read "V (during measurment)"() -> (w1219:dbl)
                    n357 = property on="squre wave" class="Bool (strict)"() -> ("Value"=w1213:bool)  [unwired: 2 in, 2 out]
                    n358 = property on="V2 applied?" class="Bool (strict)"() -> ("Value"=w1214:bool)  [unwired: 2 in, 2 out]
                    n359 = Unbundle By Name(w1223) -> ("V 1"=w1224:dbl)
                    n360 = Equal?(x=w1224, y=w1219) -> (x = y?=w1221:bool)
                    n361 = And(x=w1213, y=w1214) -> (x .and. y?=w1212:bool)
                    n362 = case shown="True" w1221 {
                      tunnel: w1223 -> [w1231 w1235]
                      tunnel: [w1231 w1235] -> w1222
                      tunnel: [w1230 w1234] -> w1220
                      tunnel: w1215 -> [w1229 w1233]
                      tunnel: w1212 -> [_ w1232]
                      frame False {
                        n363 = Unbundle By Name(w1231) -> ("V2 time"=w1227:dbl)
                        n364 = Multiply(x=1000.0, y=w1227) -> (x*y=w1228:dbl)
                        n365 = Greater Or Equal?(x=w1229, y=w1228) -> (x >= y?=w1230:bool)
                      }
                      frame True {
                        n366 = case shown="True" w1232 {
                          tunnel: w1235 -> [w1238 w1247]
                          tunnel: [w1236 w1246] -> w1234
                          tunnel: w1233 -> [w1237 w1245]
                          frame False {
                            n367 = Unbundle By Name(w1238) -> ("V1 time"=w1241:dbl)
                            n368 = Multiply(x=w1241, y=1000.0) -> (x*y=w1240:dbl)
                            n369 = Greater Or Equal?(x=w1237, y=w1240) -> (x >= y?=w1236:bool)
                          }
                          frame True {
                            n370 = Unbundle By Name(w1247) -> ("V off time"=w1243:dbl)
                            n371 = Multiply(x=w1243, y=1000.0) -> (x*y=w1244:dbl)
                            n372 = Greater Or Equal?(x=w1245, y=w1244) -> (x >= y?=w1246:bool)
                          }
                        }
                      }
                    }
                  }
                  frame "Read", Default {
                    # "Building a 1d matrix of currents"
                    n373 = property on="Use autolab?" class="Bool (strict)"() -> ("Value"=w1250:bool)  [unwired: 2 in, 2 out]
                    n374 = case shown="True" w1250 {
                      tunnel: [w1272 w1280] -> w1261
                      tunnel: [w1271 w1281] -> w1252
                      tunnel: w1249 -> [w1270 w1279]
                      tunnel: w1248 -> [_ w1282]
                      tunnel: w1248 -> [_ w1276]
                      tunnel: w1249 -> [_ w1278]
                      tunnel: w1248 -> [_ w1277]
                      frame False {
                        n375 = flat-sequence {
                          tunnel: w1270 -> [w1274]
                          tunnel: [w1273] -> w1269
                          frame #0 {
                            n376 = call "IV getcurrent.vi"("error in (no error)"=w1274) -> ("error out"=w1273:errorcluster, "value out"=w1275:dbl)  [unwired: 8 in, 1 out]
                            n377 = call "Current ranging routine (SubVI).vi"("Current"=w1275) -> ()  [unwired: 11 in]
                          }
                        }
                        n378 = call "IV getcurrent.vi"("error in (no error)"=w1269) -> ("error out"=w1271:errorcluster, "value out"=w1272:dbl)  [unwired: 8 in, 1 out]
                      }
                      frame True {
                        n379 = disable-structure shown="Enabled" {
                          disable-tunnel: w1282 -> [w1300 _]
                          disable-tunnel: [w1294 w1317] -> w1281
                          disable-tunnel: [w1292 w1326] -> w1280
                          disable-tunnel: w1279 -> [w1287 _]
                          disable-tunnel: w1278 -> [w1286 w1334]
                          disable-tunnel: w1277 -> [w1283 _]
                          disable-tunnel: w1276 -> [_ w1337]
                          frame Disabled {
                            n380 = property on="Ei" class="Ref (strict)"() -> ("Value"=w1284:refnum<k24>)  [unwired: 2 in, 2 out]
                            n381 = disable-structure shown="Disabled" {
                              disable-tunnel: w1300 -> [w1312 _]
                              disable-tunnel: [w1311 _] -> _
                              disable-tunnel: w1287 -> [w1308 _]
                              disable-tunnel: w1284 -> [w1307 _]
                              frame Disabled {
                                w1305 = 2 items=["UltraHigh_Speed", "High_Speed", "High_Stability"] ("Bandwidth")
                                w1310 = 1 items=["Off", "On"] ("CellOnOff")
                                w1306 = 0 items=["Potentiostatic", "Galvanostatic"] ("Mode")
                                n382 = property on="CurrentRange" class="Ring (strict)"() -> ("Value"=w1309:i32)  [unwired: 2 in, 2 out]
                                n383 = property class="EI"(reference=w1307, error in=w1308, "Bandwidth"=w1305, "CellOnOff"=w1310, "CurrentRange"=w1309, "Mode"=w1306, "Setpoint"=w1312) -> (error out=w1311:errorcluster)  [unwired: 1 out]
                                n384 = property on="Sampler 2" class="Ref (strict)"(error in=w1311) -> (error out=w1304:errorcluster, "Value"=w1301:refnum<k24>)  [unwired: 1 in, 1 out]
                                n385 = property class="EI"(reference=w1307, error in=w1311) -> (error out=w1302:errorcluster, "EiStatusSupportedFor"=w1303:string[])  [unwired: 1 out]
                                n386 = invoke class="Sampler" method="Sample"(reference=w1301, error in=w1304) -> ()  [unwired: 1 in, 3 out]
                                n387 = property on="EI status supported for" class="Arr (strict)"(error in=w1302, "Value"=w1303) -> ()  [unwired: 1 in, 2 out]
                              }
                              frame Enabled {
                              }
                            }
                            n388 = property class="EI"(reference=w1284, error in=w1286, "Setpoint"=w1283) -> (error out=w1285:errorcluster)  [unwired: 1 out]
                            n389 = property class="EI" props=["Bandwidth", "CurrentRange", "Mode", "Setpoint", "Current", "Potential"](reference=w1284, error in=w1285) -> (error out=w1288:errorcluster, "Bandwidth"=w1299:i32, "CurrentRange"=w1298:i32, "Mode"=w1297:i32, "Current"=w1291:dbl, "Potential"=w1290:dbl)  [unwired: 2 out]
                            n390 = property on="Bandwidth" class="Ring (strict)"("Value"=w1299) -> ()  [unwired: 2 in, 2 out]
                            n391 = property on="CurrentRange" class="Ring (strict)"("Value"=w1298) -> ()  [unwired: 2 in, 2 out]
                            n392 = property on="Mode" class="Ring (strict)"("Value"=w1297) -> ()  [unwired: 2 in, 2 out]
                            n393 = flat-sequence {
                              tunnel: [w1316] -> w1296
                              tunnel: w1291 -> [w1315]
                              tunnel: w1290 -> [w1314]
                              tunnel: [w1313] -> w1289
                              tunnel: w1288 -> [w1313]
                              frame #0 {
                                n394 = call "Range_selector.vi"("potential"=w1314, "current"=w1315) -> ("range integer"=w1316:i32)  [unwired: 9 in]
                              }
                            }
                            n395 = property class="EI"(reference=w1284, error in=w1289) -> (error out=w1295:errorcluster, "Current"=w1292:dbl, "Potential"=→"POtential PD":dbl)  [unwired: 1 out]
                            "Current PD" <- w1292
                            n396 = property class="EI"(reference=w1284, error in=w1295, "CurrentRange"=w1296) -> (error out=w1294:errorcluster)  [unwired: 1 out]
                          }
                          frame Enabled {
                            w1319 = 0 items=["Potentiostatic", "Galvanostatic"] ("Mode")
                            w1320 = 1 items=["Off", "On"] ("CellOnOff")
                            w1321 = 2 items=["UltraHigh_Speed", "High_Speed", "High_Stability"] ("Bandwidth")
                            w1327 = 1 items=["Off", "On"] ("CellOnOff")
                            w1328 = 2 items=["UltraHigh_Speed", "High_Speed", "High_Stability"] ("Bandwidth")
                            w1329 = 0 items=["Potentiostatic", "Galvanostatic"] ("Mode")
                            w1338 = 0 items=["Potentiostatic", "Galvanostatic"] ("Mode")
                            w1341 = 1 items=["Off", "On"] ("CellOnOff")
                            w1342 = 2 items=["UltraHigh_Speed", "High_Speed", "High_Stability"] ("Bandwidth")
                            n397 = property on="Sampler 2" class="Ref (strict)"() -> ("Value"=w1324:refnum<k24>)  [unwired: 2 in, 2 out]
                            n398 = property on="CurrentRange" class="Ring (strict)"() -> ("Value"=w1340:i32)  [unwired: 2 in, 2 out]
                            n399 = property on="Ei" class="Ref (strict)"() -> ("Value"=w1323:refnum<k24>)  [unwired: 2 in, 2 out]
                            n400 = call "EI (A).vi"("Sampler"=w1324, "Ei"=w1323, "CellOnOff"=w1341, "Setpoint"=w1337, "Bandwidth"=w1342, "CurrentRange"=w1340, "Mode"=w1338, "error in (no error)"=w1334, "Disable Sampler"=FALSE) -> ("Cell"=w1335:bool, "Bandwidth"=w1336:i32, "error out"=w1333:errorcluster)  [unwired: 5 in, 11 out]
                            n401 = property on="Bandwidth" class="Ring (strict)"("Value"=w1336) -> ()  [unwired: 2 in, 2 out]
                            n402 = property on="Cell on?" class="Bool (strict)"("Value"=w1335) -> ()  [unwired: 2 in, 2 out]
                            n403 = call "Sampler.vi"("error in (no error)"=w1334, "Sampler"=w1324) -> ("error out"=w1331:errorcluster)  [unwired: 7 in, 2 out]
                            n404 = Merge Errors(w1331, w1333) -> (w1332:errorcluster)
                            n405 = call "EI (A).vi"("Sampler"=w1324, "Ei"=w1323, "CellOnOff"=w1327, "Bandwidth"=w1328, "Mode"=w1329, "error in (no error)"=w1332, "Disable Sampler"=FALSE) -> ("Potential"=w1325:dbl, "Current"=w1326:dbl, "error out"=w1318:errorcluster)  [unwired: 7 in, 11 out]
                            n406 = property on="Voltage" class="DigNum (strict)"("Value"=w1325) -> ()  [unwired: 2 in, 2 out]
                            n407 = property on="current" class="DigNum (strict)"("Value"=w1326) -> ()  [unwired: 2 in, 2 out]
                            n408 = call "Range_selector.vi"("potential"=w1325, "current"=w1326) -> ("range integer"=w1322:i32)  [unwired: 9 in]
                            n409 = call "EI (A).vi"("Sampler"=w1324, "Ei"=w1323, "CellOnOff"=w1320, "Bandwidth"=w1321, "CurrentRange"=w1322, "Mode"=w1319, "error in (no error)"=w1318) -> ("error out"=w1317:errorcluster)  [unwired: 7 in, 13 out]
                          }
                        }
                      }
                    }
                    n410 = Unbundle By Name(w1254) -> ("Start time"=w1253:i32)
                    n411 = Tick Count (ms)() -> (millisecond timer value=w1251:u32)
                    n412 = Subtract(x=w1251, y=w1253) -> (x-y=w1264:u32)
                    n413 = Equal?(x=1, y=w1268) -> (x = y?=w1258:bool)
                    n414 = And(x=w1257, y=w1258) -> (x .and. y?=w1256:bool)
                    n415 = case shown="True" w1256 {
                      tunnel: [w1344 w1348] -> w1262
                      tunnel: w1263 -> [w1345 w1346]
                      tunnel: w1264 -> [w1343 w1347]
                      tunnel: [w1343 w1347] -> w1255
                      frame False {
                        n416 = Build Array (concatenate)(w1345, w1343) -> (w1344:u32[])
                      }
                      frame True {
                        n417 = Build Array (concatenate)(w1346, w1347) -> (w1348:u32[])
                      }
                    }
                    n418 = case shown="False" w1256 {
                      tunnel: [w1350 w1352] -> w1267
                      tunnel: w1266 -> [w1351 _]
                      tunnel: w1261 -> [w1349 w1353]
                      frame False {
                        # "Intensity thereafter"
                        n419 = Build Array (concatenate)(w1351, w1349) -> (w1350:dbl[])
                      }
                      frame True {
                        n420 = Build Array(w1353) -> (w1352:dbl[])
                      }
                    }
                  }
                  frame "Wait" {
                    n421 = Unbundle By Name(w1360) -> ("Sample rate"=w1361:dbl)
                    n422 = Multiply(x=w1361, y=1000.0) -> (x*y=w1363:dbl)
                    n423 = Wait (ms)(milliseconds to wait=w1363) -> ()  [unwired: 1 out]
                  }
                }
                n424 = property on="IDus not in read loop? (kinetic)" class="Bool (strict)"() -> ("Value"=w1197:bool)  [unwired: 2 in, 2 out]
                n425 = And(x=w1197, y=w1196) -> (x .and. y?=w1195:bool)
              }
              n426 = case shown="True" w892 {
                tunnel: [w931 w1021] -> w908
                tunnel: [w930 w1023] -> w907
                tunnel: [w919 w1020] -> w906
                tunnel: w900 -> [w929 w1022]
                tunnel: w883 -> [w928 w1026]
                tunnel: w898 -> [w923 w1027]
                tunnel: w895 -> [w922 w1025]
                tunnel: w880 -> [w921 w1024]
                tunnel: w884 -> [_ w1019]
                tunnel: w882 -> [_ w1018]
                frame False {
                  n427 = Unbundle By Name(w921) -> ("Continous strobe delay"=w927:i32, "Integration time"=w926:i32)  [unwired: 1 out]
                  n428 = call "Initalise spectrometer.vi"("Continous strobe delay"=w927, "Enter the \nInetegration Time"=w926) -> ("Wrapper Out"=w920:u32, "ContinuousStrobe Out"=w925:u32, "WL Values"=w924:dbl[])  [unwired: 7 in]
                  "ContinuousStrobe Out" <- w925
                  "Wrapper Out" <- w920
                  "WL Values" <- w924
                  n429 = while {
                    shift-right: [w948] -> _
                    shift-left: w921 -> [w949]
                    shift-right: [w940] -> _
                    shift-left: OSPEC-enum."Wait" -> [w950]
                    shift-right: [w946] -> w919
                    shift-left: w922 -> [w945]
                    shift-right: [w938] -> w930
                    shift-left: w923 -> [w944]
                    shift-right: [w943] -> w931
                    shift-left: w929 -> [w942]
                    tunnel: w928 -> [w939]
                    tunnel: w920 -> [w937]
                    tunnel: [w936] -> _
                    tunnel: w925 -> [w935]
                    tunnel: w924 -> [w934]
                    tunnel: [w933] -> _
                    i -> [w941]
                    stop <- w947 stop-if-true
                    n430 = case shown="\"Read\", Default" w950 {
                      tunnel: w949 -> [w959 w975 w1014]
                      tunnel: [w958 w975 w1014] -> w948
                      tunnel: [w956 FALSE FALSE] -> w947
                      tunnel: [w960 w994 w1012] -> w946
                      tunnel: w945 -> [w960 w993 w1012]
                      tunnel: w941 -> [_ w988 _]
                      tunnel: [w951 w981 w1007] -> w938
                      tunnel: w944 -> [w951 w992 w1007]
                      tunnel: [w957 w983 w1011] -> w943
                      tunnel: w942 -> [w957 _ w1011]
                      tunnel: [OSPEC-enum."Wait" OSPEC-enum."Check exit" OSPEC-enum."Read"] -> w940
                      tunnel: w939 -> [w954 w987 _]
                      tunnel: w937 -> [w952 w979 w1008]
                      tunnel: [w953 w980 w1009] -> w936
                      tunnel: w935 -> [w953 w980 w1009]
                      tunnel: w934 -> [_ w978 _]
                      tunnel: [w952 w979 w1008] -> w933
                      frame "Check exit" {
                        n431 = case shown="False" w954 {
                          tunnel: w959 -> [w966 w972]
                          tunnel: [w966 w972] -> w958
                          tunnel: w957 -> [w964 w970]
                          tunnel: [w965 w971] -> w956
                          frame False {
                            n432 = Unbundle By Name(w966) -> ("V2 time"=w963:dbl)
                            n433 = Multiply(x=w963, y=1000.0) -> (x*y=w961:dbl)
                            n434 = Greater Or Equal?(x=w964, y=w961) -> (x >= y?=w965:bool)
                          }
                          frame True {
                            n435 = Unbundle By Name(w972) -> ("V1 time"=w969:dbl)
                            n436 = Multiply(x=w969, y=1000.0) -> (x*y=w967:dbl)
                            n437 = Greater Or Equal?(x=w970, y=w967) -> (x >= y?=w971:bool)
                          }
                        }
                      }
                      frame "Read", Default {
                        # "Check here to see if DIM t + 1 and DIM WL match"
                        n438 = Tick Count (ms)() -> (millisecond timer value=w973:u32)
                        n439 = call "Wrapper_getSpectrum.vi"("Index"=0, "Wrapper"=w979) -> ("Spectrum Values"=w977:dbl[])  [unwired: 1 out]
                        n440 = Unbundle By Name(w975) -> ("Start time"=w974:i32)
                        n441 = Subtract(x=w973, y=w974) -> (x-y=w984:u32)
                        n442 = Bundle("WL Values"=w978, "Spectrum Values"=w977) -> (→"?":T5)  [unwired: 1 in]
                        n443 = Equal?(x=w988, y=1.0) -> (x = y?=w986:bool)
                        n444 = And(x=w987, y=w986) -> (x .and. y?=w985:bool)
                        n445 = case shown="True" w985 {
                          tunnel: [w997 w998] -> w981
                          tunnel: w992 -> [w996 _]
                          tunnel: w977 -> [w995 w1000]
                          tunnel: w978 -> [_ w999]
                          frame False {
                            # "Intensity thereafter"
                            n446 = Build Array (concatenate)(w996, w995) -> (w997:dbl[][])
                          }
                          frame True {
                            n447 = Build Array(w999, w1000) -> (w998:dbl[][])
                          }
                        }
                        n448 = case shown="True" w985 {
                          tunnel: [w1003 w1006] -> w994
                          tunnel: w993 -> [w1002 w1005]
                          tunnel: w984 -> [w1001 w1004]
                          tunnel: [w1001 w1004] -> w983
                          frame False {
                            n449 = Build Array (concatenate)(w1002, w1001) -> (w1003:u32[])
                          }
                          frame True {
                            n450 = Build Array (concatenate)(w1005, w1004) -> (w1006:u32[])
                          }
                        }
                      }
                      frame "Wait" {
                        n451 = Unbundle By Name(w1014) -> ("Sample rate"=w1015:dbl)
                        n452 = Multiply(x=w1015, y=1000.0) -> (x*y=w1017:dbl)
                        n453 = Wait (ms)(milliseconds to wait=w1017) -> ()  [unwired: 1 out]
                      }
                    }
                  }
                }
                frame True {
                  n454 = while {
                    shift-right: [w1041] -> w1021
                    shift-left: w1022 -> [w1042]
                    shift-right: [w1034] -> _
                    shift-left: OSPEC-enum."Wait" -> [w1043]
                    shift-right: [w1040] -> w1020
                    shift-left: w1025 -> [w1039]
                    shift-right: [w1032] -> w1023
                    shift-left: w1027 -> [w1038]
                    shift-right: [w1037] -> _
                    shift-left: w1024 -> [w1036]
                    tunnel: w1026 -> [w1033]
                    tunnel: w1019 -> [w1030]
                    tunnel: w1018 -> [w1029]
                    i -> [w1035]
                    stop <- w1031 stop-if-true
                    n455 = case shown="\"Read\", Default" w1043 {
                      tunnel: w1042 -> [w1052 _ w1191]
                      tunnel: [w1051 w1079 w1191] -> w1041
                      tunnel: [w1049 FALSE FALSE] -> w1031
                      tunnel: [w1053 w1080 w1189] -> w1040
                      tunnel: w1039 -> [w1053 w1085 w1189]
                      tunnel: w1035 -> [_ w1089 _]
                      tunnel: w1038 -> [w1047 w1083 w1185]
                      tunnel: [w1050 w1078 w1187] -> w1037
                      tunnel: w1036 -> [w1050 w1078 w1187]
                      tunnel: [OSPEC-enum."Wait" OSPEC-enum."Check exit" OSPEC-enum."Read"] -> w1034
                      tunnel: w1033 -> [_ w1084 _]
                      tunnel: [w1047 w1081 w1185] -> w1032
                      tunnel: w1030 -> [w1046 _ _]
                      tunnel: w1029 -> [w1045 _ _]
                      frame "Check exit" {
                        n456 = case shown="True" w1046 {
                          tunnel: w1052 -> [w1055 w1064]
                          tunnel: [w1055 w1063] -> w1051
                          tunnel: w1050 -> [w1054 w1062]
                          tunnel: [w1056 w1061] -> w1049
                          tunnel: w1045 -> [_ w1060]
                          frame False {
                            n457 = Unbundle By Name(w1054) -> ("V2 time"=w1057:dbl)
                            n458 = Multiply(x=w1057, y=1000.0) -> (x*y=w1058:dbl)
                            n459 = Greater Or Equal?(x=w1055, y=w1058) -> (x >= y?=w1056:bool)
                          }
                          frame True {
                            n460 = case shown="False" w1060 {
                              tunnel: w1064 -> [w1066 w1071]
                              tunnel: [w1066 w1071] -> w1063
                              tunnel: w1062 -> [w1065 w1072]
                              tunnel: [w1070 w1076] -> w1061
                              frame False {
                                n461 = Unbundle By Name(w1065) -> ("V1 time"=w1067:dbl)
                                n462 = Multiply(x=w1067, y=1000.0) -> (x*y=w1068:dbl)
                                n463 = Greater Or Equal?(x=w1066, y=w1068) -> (x >= y?=w1070:bool)
                              }
                              frame True {
                                n464 = Unbundle By Name(w1072) -> ("V off time"=w1073:dbl)
                                n465 = Multiply(x=w1073, y=1000.0) -> (x*y=w1074:dbl)
                                n466 = Greater Or Equal?(x=w1071, y=w1074) -> (x >= y?=w1076:bool)
                              }
                            }
                          }
                        }
                      }
                      frame "Read", Default {
                        n467 = Unbundle By Name(w1078) -> ("Start time"=w1077:i32)
                        n468 = property on="Number of scans in kinetic cycle" class="DigNum (strict)"() -> ("Value"=w1088:i32)  [unwired: 2 in, 2 out]
                        n469 = Tick Count (ms)() -> (millisecond timer value=w1086:u32)
                        n470 = Subtract(x=w1086, y=w1077) -> (x-y=w1079:u32)
                        n471 = call "GetDetector.vi"() -> ("xpixels"=w1087:i32)  [unwired: 4 in, 3 out]
                        n472 = Equal?(x=w1089, y=1.0) -> (x = y?=w1082:bool)
                        n473 = stacked-sequence {
                          seq-local: [_ _ _ _ _ _ _ _ _ _ w1123 _] -> [_ _ _ _ _ _ _ _ _ _ _ w1144]
                          seq-local: [_ _ _ _ _ _ _ _ w1108 _ _ _] -> [_ _ _ _ _ _ _ _ _ _ _ w1142]
                          seq-local: [_ _ _ _ _ _ _ _ _ _ w1122 _] -> [_ _ _ _ _ _ _ _ _ _ _ w1143]
                          tunnel: [_ _ _ _ _ _ _ _ _ _ _ w1137] -> w1081
                          tunnel: [_ _ _ _ _ _ _ _ _ _ _ w1138] -> w1080
                          tunnel: w1088 -> [_ _ _ _ _ w1101 _ _ _ _ w1119 w1136]
                          tunnel: w1079 -> [_ _ _ _ _ _ _ _ _ _ _ w1139]
                          tunnel: w1087 -> [_ w1094 _ _ _ _ _ _ _ _ _ _]
                          tunnel: w1077 -> [_ _ _ _ _ _ _ _ w1107 _ w1121 _]
                          tunnel: w1085 -> [_ _ _ _ _ _ _ _ _ _ _ w1135]
                          tunnel: w1084 -> [_ _ _ _ _ _ _ _ _ _ _ w1134]
                          tunnel: w1083 -> [_ _ _ _ _ _ _ _ _ _ _ w1133]
                          tunnel: w1082 -> [_ _ _ _ _ _ _ _ _ _ _ w1132]
                          frame #0 {
                            w1093 = u16 3  # AcquisitionMode
                            n474 = call "SetAcquisitionMode.vi"("mode"=w1093) -> ()  [unwired: 1 in, 2 out]
                          }
                          frame #1 {
                            w1095 = u16 0  # ReadMode
                            n475 = property on="xpixels" class="DigNum (strict)"("Value"=w1094) -> ()  [unwired: 2 in, 2 out]
                            n476 = call "SetReadMode.vi"("mode"=w1095) -> ()  [unwired: 1 in, 2 out]
                          }
                          frame #2 {
                            n477 = call "SetTriggerMode.vi"("mode"=TriggerMode_mode_typedef."Internal") -> ()  [unwired: 1 in, 2 out]
                          }
                          frame #3 {
                            n478 = property on="Exposure time (s)" class="DigNum (strict)"() -> ("Value"=w1097:dbl)  [unwired: 2 in, 2 out]
                            n479 = call "SetExposureTime.vi"("time"=w1097) -> ()  [unwired: 1 in, 2 out]
                          }
                          frame #4 {
                            n480 = call "GetNumberVSSpeeds.vi"() -> ("number"=w1100:i32)  [unwired: 3 in, 2 out]
                            n481 = Subtract(x=w1100, y=1) -> (x-y=w1098:i32)
                            n482 = call "SetVSSpeed.vi"("index"=w1098) -> ()  [unwired: 1 in, 2 out]
                          }
                          frame #5 {
                            n483 = call "SetNumberKinetics.vi"("number"=w1101) -> ()  [unwired: 1 in, 2 out]
                          }
                          frame #6 {
                            w1104 = 0  # Auto Shutter
                            n484 = call "SetShutter.vi"("type"="Shutter opens on TTL", "mode"=w1104, "closingtime"="Shutter open and close time", "openingtime"="Shutter open and close time") -> ()  [unwired: 10 in, 2 out]
                          }
                          frame #7 {
                            # "Meybe delete the exposure time insupt here"
                            n485 = property on="Exposure time (s)" class="DigNum (strict)"() -> ("Value"=w1105:dbl)  [unwired: 2 in, 2 out]
                            n486 = call "GetAcquisitionTimings.vi"("exposure input"=w1105) -> ("exposure"=w1106:sgl)  [unwired: 10 in, 4 out]
                            n487 = property on="Calculated exposure time" class="DigNum (strict)"("Value"=w1106) -> ()  [unwired: 2 in, 2 out]
                          }
                          frame #8 {
                            n488 = flat-sequence {
                              tunnel: [w1110] -> w1108
                              tunnel: w1107 -> [w1109]
                              frame #0 {
                                n489 = Tick Count (ms)() -> (millisecond timer value=w1111:u32)
                                n490 = Subtract(x=w1111, y=w1109) -> (x-y=w1110:u32)
                                "Time before the start of current aquisition (ms)" <- w1110
                              }
                              frame #1 {
                                n491 = call "StartAcquisition.vi"() -> ("DLL error code"=w1112:u32)  [unwired: 2 in, 1 out]
                                n492 = property on="Start Aquisition return code" class="DigNum (strict)"("Value"=w1112) -> ()  [unwired: 2 in, 2 out]
                              }
                            }
                          }
                          frame #9 {
                            n493 = while {
                              stop <- w1116 continue-if-true
                              w1117 = u16 72  # DRV ACQUIRING
                              n494 = call "GetStatus.vi"() -> ("DLL error code"=w1114:u32, "status"=w1115:T18)  [unwired: 3 in, 1 out]
                              n495 = property on="Get status return code" class="DigNum (strict)"("Value"=w1114) -> ()  [unwired: 2 in, 2 out]
                              n496 = Equal?(x=w1115, y=w1117) -> (x = y?=w1116:bool)
                              "IDus not in read loop? (kinetic)" <- FALSE
                            }
                          }
                          frame #10 {
                            n497 = flat-sequence {
                              tunnel: [w1124] -> w1122
                              tunnel: w1121 -> [w1125]
                              tunnel: [w1131] -> w1123
                              tunnel: w1120 -> [w1127]
                              frame #0 {
                                n498 = Tick Count (ms)() -> (millisecond timer value=w1126:u32)
                                n499 = Subtract(x=w1126, y=w1125) -> (x-y=w1124:u32)
                                "Time  after the aquisition (before fetch data), (ms)" <- w1124
                              }
                              frame #1 {
                                n500 = call "GetAcquiredData.vi"("size"=w1127) -> ("DLL error code"=w1128:u32, "array"=w1131:i32[])  [unwired: 2 in, 1 out]
                                n501 = Equal?(x=20002 ("DRV_SUCCESS"), y=w1128) -> (x = y?=→"Get aqisition ok? (kinetic mode)":bool)
                                n502 = property on="get aquired data return code" class="DigNum (strict)"("Value"=w1128) -> ()  [unwired: 2 in, 2 out]
                              }
                            }
                            n503 = Multiply(x=1024, y=w1119) -> (x*y=w1120:i32)
                          }
                          frame #11 {
                            n504 = Subtract(x=w1143, y=w1142) -> (x-y=w1141:u32)
                            n505 = Divide(x=w1141, y=w1136) -> (x/y=w1140:dbl)
                            n506 = for {
                              N: w1136 -> [_]
                              tunnel: w1144 -> [w1162]
                              tunnel: w1140 -> [w1160]
                              tunnel: w1139 -> [w1157]
                              shift-right: [w1155] -> w1137
                              shift-left: w1133 -> [w1154]
                              shift-right: [w1147] -> w1138
                              shift-left: w1135 -> [w1152]
                              tunnel: w1134 -> [w1150]
                              tunnel: w1132 -> [w1148]
                              i -> [w1146]
                              w1156 = 1024 ("x")
                              n507 = Equal To 0?(x=w1146) -> (x = 0?=w1145:bool)
                              n508 = Multiply(x=w1146, y=w1160) -> (x*y=w1159:dbl)
                              n509 = Multiply(x=w1156, y=w1146) -> (x*y=w1161:i32)
                              n510 = Add(x=w1159, y=w1157) -> (x+y=w1153:dbl)
                              n511 = Array Subset(array=w1162, index=w1161, length=w1156) -> (w1158:i32[])
                              n512 = And(x=w1145, y=w1148) -> (x .and. y?=w1149:bool)
                              n513 = And(x=w1150, y=w1149) -> (x .and. y?=w1151:bool)
                              n514 = case shown="False" w1151 {
                                tunnel: w1158 -> [w1163 w1176]
                                tunnel: [w1168 w1179] -> w1155
                                tunnel: w1154 -> [w1169 _]
                                tunnel: w1153 -> [w1166 w1181]
                                tunnel: [w1165 w1180] -> w1147
                                tunnel: w1152 -> [w1167 _]
                                tunnel: w1145 -> [w1164 _]
                                frame False {
                                n515 = case shown="True" w1164 {
                                tunnel: w1163 -> [_ w1172]
                                frame False {
                                }
                                frame True {
                                n516 = for {
                                N: 1023 -> [_]
                                tunnel: [w1174] -> _ mode=indexing
                                tunnel: [w1174] -> w1171 mode=indexing
                                i -> [w1175]
                                n517 = Increment(x=w1175) -> (x+1=w1174:i32)
                                }
                                n518 = Bundle(w1171, w1172) -> (w1170:cluster{i32[], i32[]})  [unwired: 1 in]
                                n519 = property class="XYGraph (strict)"("Value"=w1170) -> ()  [unwired: 2 in, 2 out]
                                }
                                }
                                n520 = Build Array (concatenate)(w1169, w1163) -> (w1168:dbl[][])
                                n521 = Build Array (concatenate)(w1167, w1166) -> (w1165:dbl[])
                                }
                                frame True {
                                n522 = for {
                                N: 1023 -> [_]
                                tunnel: [w1183] -> w1177 mode=indexing
                                i -> [w1184]
                                n523 = Increment(x=w1184) -> (x+1=w1183:i32)
                                }
                                n524 = Bundle(w1177, w1176) -> (w1178:cluster{i32[], i32[]})  [unwired: 1 in]
                                n525 = Build Array(w1181) -> (w1180:dbl[])
                                n526 = Build Array(w1177, w1176) -> (w1179:i32[][])
                                n527 = property class="XYGraph (strict)"("Value"=w1178) -> ()  [unwired: 2 in, 2 out]
                                }
                              }
                            }
                          }
                        }
                      }
                      frame "Wait" {
                        n528 = Unbundle By Name(w1187) -> ("Sample rate"=w1186:dbl)
                        n529 = Multiply(x=w1186, y=1000.0) -> (x*y=w1193:dbl)
                        n530 = Wait (ms)(milliseconds to wait=w1193) -> ()  [unwired: 1 out]
                      }
                    }
                    n531 = case shown="True" w1031 {
                      frame False {
                      }
                      frame True {
                        n532 = property on="IDus not in read loop? (kinetic)" class="Bool (strict)"("Value"=TRUE ("IDus not in read loop? (kinetic)")) -> ()  [unwired: 2 in, 2 out]
                      }
                    }
                  }
                }
              }
              n533 = Bundle By Name(cluster=w880, "Time for spectrum measurment"=w906, "Time elapsed"=w908, "Spectrum"=w907) -> (w903:T11)
              n534 = Bundle By Name(cluster=w903, "Time for I measurment"=w905, "Current array"=w891) -> (w904:T11)
              n535 = local read "V (during measurment)"() -> (w910:dbl)
              n536 = property on="V2 applied?" class="Bool (strict)"() -> ("Value"=w890:bool)  [unwired: 2 in, 2 out]
              n537 = Unbundle By Name(w903) -> ("V 1"=w911:dbl)
              n538 = Equal?(x=w911, y=w910) -> (x = y?=w912:bool)
              n539 = And(x=w890, y="squre wave") -> (x .and. y?=w889:bool)
              n540 = case shown="True" w912 {
                tunnel: [w1365 w1369] -> w913
                tunnel: w889 -> [_ w1368]
                tunnel: "squre wave" -> [w1364 _]
                frame False {
                  n541 = case shown="True" w1364 {
                    tunnel: [OSSPEC."Read Potential and spectrum" OSSPEC."Apply V1"] -> w1365
                    frame False {
                    }
                    frame True {
                    }
                  }
                }
                frame True {
                  n542 = case shown="True" w1368 {
                    tunnel: [OSSPEC."Apply V2" OSSPEC."End measurment"] -> w1369
                    frame False {
                    }
                    frame True {
                    }
                  }
                }
              }
            }
            frame "Reinitialise Cell" {
              # "this state is no longer used as it adds a 1-300 ms delay before the spectrum is measured as the mode is shifted"
              n543 = flat-sequence {
                tunnel: w1378 -> [w1382]
                tunnel: [w1381] -> w1373
                tunnel: w1373 -> [w1385]
                tunnel: [w1384] -> w1372
                tunnel: [w1386] -> w1377
                tunnel: w1372 -> [w1386]
                frame #0 {
                  n544 = To Long Integer(number=T17."IStat4EL" ("Configuration")) -> (32bit integer=w1380:i32)
                  n545 = call "IV setconnectionmode.vi"("error in (no error)"=w1382, "value"=w1380) -> ("error out"=w1381:errorcluster)  [unwired: 7 in, 2 out]
                }
                frame #1 {
                  n546 = call "IV setcurrent.vi"("error in (no error)"=w1385, "value"=0.0) -> ("error out"=w1384:errorcluster)  [unwired: 7 in, 2 out]
                }
                frame #2 {
                }
              }
              n547 = Unbundle By Name(w1374) -> ()  [unwired: 3 out]
            }
            frame "Apply V1" {
              n548 = property on="Use autolab?" class="Bool (strict)"() -> ("Value"=w1388:bool)  [unwired: 2 in, 2 out]
              n549 = flat-sequence {
                tunnel: w1396 -> [w1402]
                tunnel: w1395 -> [w1401]
                tunnel: [w1400] -> w1390
                tunnel: [w1399] -> w1389
                tunnel: w1388 -> [w1398]
                tunnel: [w1397] -> w1387
                tunnel: w1396 -> [w1443]
                tunnel: w1390 -> [w1441]
                tunnel: [w1442] -> w1392
                tunnel: [w1437] -> w1391
                tunnel: w1389 -> [w1436]
                tunnel: w1388 -> [w1435]
                tunnel: w1387 -> [w1434]
                frame #0 {
                  n550 = case shown="True" w1398 {
                    tunnel: w1402 -> [w1408 w1425]
                    tunnel: w1401 -> [w1407 _]
                    tunnel: [w1406 w1417] -> w1400
                    tunnel: [w1404 w1424] -> w1399
                    tunnel: [refnum<k24> refnum ("Value") w1421] -> w1397
                    frame False {
                      n551 = Unbundle By Name(w1408) -> ("V 1"=w1406:dbl)
                      n552 = Absolute Value(x=w1406) -> (abs(x)=w1410:dbl)
                      n553 = local write "V (during measurment)"(w1406) -> ()
                      n554 = Greater?(x=w1410, y=3.0) -> (0:w1409:bool)
                      n555 = case shown="False" w1409 {
                        tunnel: [w1411 w1413] -> w1404
                        tunnel: w1407 -> [w1411 w1412]
                        frame False {
                        }
                        frame True {
                          # "abort if E >3 V"
                          n556 = call "IV setcellon.vi"("error in (no error)"=w1412, "cellon"=0) -> ("error out"=w1415:errorcluster)  [unwired: 7 in, 2 out]
                          n557 = call "IV close.vi"("error in (no error)"=w1415) -> ("error out"=w1413:errorcluster)  [unwired: 9 in, 1 out]
                          n558 = call "Display Message to User3"("error in (no error)"=w1413) -> ("OK"=w1416:bool)  [unwired: 9 in, 1 out]
                          n559 = Stop(stop? (T)=w1416) -> ()
                        }
                      }
                    }
                    frame True {
                      w1431 = 1 items=["Off", "On"] ("CellOnOff")
                      n560 = property on="Ei" class="Ref (strict)"() -> ("Value"=w1421:refnum<k24>)  [unwired: 2 in, 2 out]
                      n561 = property on="Sampler 2" class="Ref (strict)"() -> ("Value"=w1427:refnum<k24>)  [unwired: 2 in, 2 out]
                      n562 = property class="EI" props=["EiStatusSupportedFor"](reference=w1421) -> (error out=w1423:errorcluster)  [unwired: 1 in, 2 out]
                      n563 = property class="EI" props=["Bandwidth", "CurrentRange", "Mode", "Potential", "Current"](reference=w1421) -> (error out=w1429:errorcluster, "Potential"=w1433:dbl, "Current"=w1432:dbl)  [unwired: 1 in, 4 out]
                      n564 = invoke class="Sampler" method="Sample"(reference=w1427) -> (error out=w1422:errorcluster)  [unwired: 2 in, 2 out]
                      n565 = Unbundle By Name(w1425) -> ("V 1"=w1417:dbl)
                      n566 = call "Range_selector.vi"("potential"=w1433, "current"=w1432) -> ("range integer"=w1430:i32)  [unwired: 9 in]
                      n567 = property class="EI"(reference=w1421, error in=w1429, "CellOnOff"=w1431, "CurrentRange"=w1430) -> (error out=w1428:errorcluster)  [unwired: 1 out]
                      n568 = call "P_Stat_Status1.vi"("error in (no error)"=w1428, ".NET Refnum in"=w1421) -> ("error out"=w1426:errorcluster, "PotentialOverload"=w1418:bool, "CurrentOverload"=w1420:bool, "Cell"=w1419:bool)  [unwired: 3 in, 3 out]
                      n569 = Merge Errors(w1426, w1423, w1422) -> (w1424:errorcluster)
                      n570 = property on="V (during measurment)" class="DigNum (strict)"("Value"=w1417) -> ()  [unwired: 2 in, 2 out]
                      n571 = property on="Cell on?" class="Bool (strict)"("Value"=w1419) -> ()  [unwired: 2 in, 2 out]
                      n572 = property on="PotentialOverload" class="Bool (strict)"("Value"=w1418) -> ()  [unwired: 2 in, 2 out]
                      n573 = property on="CurrentOverload" class="Bool (strict)"("Value"=w1420) -> ()  [unwired: 2 in, 2 out]
                    }
                  }
                }
                frame #1 {
                  n574 = property on="squre wave" class="Bool (strict)"() -> ("Value"=w1439:bool)  [unwired: 2 in, 2 out]
                  n575 = property on="V2 applied?" class="Bool (strict)"() -> ("Value"=w1440:bool)  [unwired: 2 in, 2 out]
                  n576 = case shown="True" w1435 {
                    tunnel: w1441 -> [w1446 w1449]
                    tunnel: [w1445 w1448] -> w1437
                    tunnel: w1436 -> [w1444 w1450]
                    tunnel: w1434 -> [_ w1447]
                    frame False {
                      n577 = call "IV setpotential.vi"("error in (no error)"=w1444, "value"=w1446) -> ("error out"=w1445:errorcluster)  [unwired: 7 in, 2 out]
                    }
                    frame True {
                      n578 = property class="EI"(reference=w1447, error in=w1450, "Setpoint"=w1449) -> (error out=w1448:errorcluster)  [unwired: 1 out]
                    }
                  }
                  n579 = And(x=w1439, y=w1440) -> (x .and. y?=w1438:bool)
                  n580 = case shown="False" w1438 {
                    tunnel: w1443 -> [w1454 w1455]
                    tunnel: [w1453 w1455] -> w1442
                    frame False {
                      n581 = Tick Count (ms)() -> (millisecond timer value=w1451:u32)
                      n582 = Bundle By Name(cluster=w1454, "Start time"=w1451, "Time elapsed"=0) -> (w1453:T11)
                    }
                    frame True {
                    }
                  }
                }
              }
            }
            frame "Apply V2" {
              n583 = Tick Count (ms)() -> (millisecond timer value=w1463:u32)
              n584 = flat-sequence {
                tunnel: w1458 -> [w1476]
                tunnel: [w1477] -> w1469
                tunnel: w1468 -> [w1475]
                tunnel: [w1470] -> w1465
                tunnel: [w1474] -> w1464
                tunnel: w1463 -> [w1474]
                tunnel: w1458 -> [w1473]
                tunnel: [w1472] -> w1457
                tunnel: [w1471] -> w1456
                tunnel: w1469 -> [w1513]
                tunnel: w1465 -> [w1512]
                tunnel: w1464 -> [w1511]
                tunnel: [w1511] -> w1461
                tunnel: [w1510] -> w1459
                tunnel: w1457 -> [w1508]
                tunnel: w1456 -> [w1507]
                frame #0 {
                  n585 = property on="Use autolab?" class="Bool (strict)"() -> ("Value"=w1472:bool)  [unwired: 2 in, 2 out]
                  n586 = Unbundle By Name(w1476) -> ("V 2"=w1470:dbl)
                  n587 = Absolute Value(x=w1470) -> (abs(x)=w1480:dbl)
                  n588 = Greater?(x=w1480, y=3.0) -> (0:w1478:bool)
                  n589 = local write "V (during measurment)"(w1470) -> ()
                  n590 = case shown="True" w1472 {
                    tunnel: w1478 -> [w1484 _]
                    tunnel: [w1483 w1497] -> w1477
                    tunnel: w1475 -> [w1482 _]
                    tunnel: w1473 -> [_ _]
                    tunnel: [refnum<k24> refnum ("Value") w1496] -> w1471
                    tunnel: w1470 -> [_ w1494]
                    frame False {
                      n591 = case shown="True" w1484 {
                        tunnel: [w1485 w1487] -> w1483
                        tunnel: w1482 -> [w1485 w1486]
                        frame False {
                        }
                        frame True {
                          # "abort if E >3 V"
                          n592 = call "IV setcellon.vi"("error in (no error)"=w1486, "cellon"=0) -> ("error out"=w1489:errorcluster)  [unwired: 7 in, 2 out]
                          n593 = call "IV close.vi"("error in (no error)"=w1489) -> ("error out"=w1487:errorcluster)  [unwired: 9 in, 1 out]
                          n594 = call "Display Message to User4"("error in (no error)"=w1487) -> ("OK"=w1490:bool)  [unwired: 9 in, 1 out]
                          n595 = Stop(stop? (T)=w1490) -> ()
                        }
                      }
                    }
                    frame True {
                      w1504 = 1 items=["Off", "On"] ("CellOnOff")
                      n596 = property on="Ei" class="Ref (strict)"() -> ("Value"=w1496:refnum<k24>)  [unwired: 2 in, 2 out]
                      n597 = property on="Sampler 2" class="Ref (strict)"() -> ("Value"=w1498:refnum<k24>)  [unwired: 2 in, 2 out]
                      n598 = property class="EI"(reference=w1496) -> (error out=w1495:errorcluster, "EiStatusSupportedFor"=w1493:string[])  [unwired: 1 in, 1 out]
                      n599 = property class="EI" props=["Bandwidth", "CurrentRange", "Mode", "Potential", "Current"](reference=w1496) -> (error out=w1502:errorcluster, "Potential"=w1506:dbl, "Current"=w1505:dbl)  [unwired: 1 in, 4 out]
                      n600 = invoke class="Sampler" method="Sample"(reference=w1498) -> (error out=w1499:errorcluster)  [unwired: 2 in, 2 out]
                      n601 = call "Range_selector.vi"("potential"=w1506, "current"=w1505) -> ("range integer"=w1503:i32)  [unwired: 9 in]
                      n602 = property class="EI"(reference=w1496, error in=w1502, "CellOnOff"=w1504, "CurrentRange"=w1503, "Setpoint"=w1494) -> (error out=w1501:errorcluster)  [unwired: 1 out]
                      n603 = property on="EI status supported for" class="Arr (strict)"("Value"=w1493) -> ()  [unwired: 2 in, 2 out]
                      n604 = call "P_Stat_Status1.vi"("error in (no error)"=w1501, ".NET Refnum in"=w1496) -> ("error out"=w1500:errorcluster, "PotentialOverload"=w1491:bool, "CurrentOverload"=w1492:bool)  [unwired: 3 in, 4 out]
                      n605 = property on="CurrentOverload" class="Bool (strict)"("Value"=w1492) -> ()  [unwired: 2 in, 2 out]
                      n606 = Merge Errors(w1500, w1495, w1499) -> (w1497:errorcluster)
                      n607 = property on="PotentialOverload" class="Bool (strict)"("Value"=w1491) -> ()  [unwired: 2 in, 2 out]
                    }
                  }
                }
                frame #1 {
                  n608 = case shown="True" w1508 {
                    tunnel: w1513 -> [w1516 w1519]
                    tunnel: w1512 -> [w1515 w1517]
                    tunnel: [w1514 w1518] -> w1510
                    tunnel: w1507 -> [_ w1520]
                    frame False {
                      n609 = call "IV setpotential.vi"("error in (no error)"=w1516, "value"=w1515) -> ("error out"=w1514:errorcluster)  [unwired: 7 in, 2 out]
                    }
                    frame True {
                      n610 = property class="EI"(reference=w1520, error in=w1519, "Setpoint"=w1517) -> (error out=w1518:errorcluster)  [unwired: 1 out]
                    }
                  }
                  "V2 applied?" <- TRUE ("V2 applied")
                }
              }
              n611 = Tick Count (ms)() -> (millisecond timer value=w1460:u32)
              n612 = Subtract(x=w1460, y=w1461) -> (x-y=→"Time taken to apply V2":u32)
              n613 = Unbundle By Name(w1458) -> ()  [unwired: 3 out]
            }
            frame "End measurment" {
              w1530 = ext 0.00099999999999999999996
              n614 = Unbundle By Name(w1524) -> ("Time for spectrum measurment"=w1526:i32[], "Spectrum"=w1543:dbl[][])
              n615 = Unbundle By Name(w1524) -> ("Current array"=w1537:dbl[], "Time for I measurment"=w1532:i32[])
              n616 = Unbundle By Name(w1524) -> ("Time for E measurment"=w1529:i32[], "Potential array"=w1538:dbl[])
              n617 = Multiply(x=w1526, y=ext 0.00099999999999999999996) -> (x*y=w1525:ext[])
              n618 = Insert Into Array(array=w1525, index=0, new element=0 ("new element/subarray")) -> (w1541:ext[])
              n619 = Multiply(x=w1530, y=w1529) -> (x*y=w1528:ext[])
              n620 = Multiply(x=w1532, y=w1530) -> (x*y=w1531:ext[])
              n621 = Build Array(w1531, w1537) -> (w1536:ext[][])
              n622 = Build Array(w1528, w1538) -> (w1534:ext[][])
              n623 = Insert Into Array(array=w1543, index (col)=0 ("disabled index (col)"), new element=w1541) -> (w1540:dbl[][])  [unwired: 1 in]
              n624 = Transpose 2D Array(2D array=w1534) -> (transposed array=w1533:ext[][])
              n625 = Transpose 2D Array(2D array=w1536) -> (transposed array=w1535:ext[][])
              n626 = call "Write-OSP-E-t.vi"("Init cluster"=w1524, "Array"=w1533) -> ()  [unwired: 10 in]
              n627 = Transpose 2D Array(2D array=w1540) -> (transposed array=w1539:dbl[][])
              n628 = call "Write-OSP-J-t.vi"("Init cluster"=w1524, "Array"=w1535) -> ()  [unwired: 10 in]
              n629 = call "Write-OSP-SP.vi"("Init cluster"=w1524, "Array"=w1539) -> ()  [unwired: 10 in]
              n630 = property on="T reached?" class="Bool (strict)"("Value"=FALSE ("T reached?")) -> ()  [unwired: 2 in, 2 out]
              n631 = Unbundle By Name(w1524) -> ("Default\n potential"=w1521:dbl)
              n632 = property on="Use autolab?" class="Bool (strict)"() -> ("Value"=w1522:bool)  [unwired: 2 in, 2 out]
              n633 = case shown="True" w1522 {
                tunnel: w1521 -> [w1552 w1568]
                tunnel: w1549 -> [w1551 w1567]
                tunnel: [w1550 w1566] -> w1546
                frame False {
                  n634 = flat-sequence {
                    tunnel: w1551 -> [w1556]
                    tunnel: [w1555] -> w1554
                    tunnel: w1552 -> [w1561]
                    tunnel: w1554 -> [w1560]
                    tunnel: [w1559] -> w1553
                    tunnel: w1553 -> [w1563]
                    tunnel: [w1562] -> w1550
                    frame #0 {
                      n635 = To Long Integer(number=T17."EStat4EL" ("Configuration")) -> (32bit integer=w1558:i32)
                      n636 = call "IV setconnectionmode.vi"("error in (no error)"=w1556, "value"=w1558) -> ("error out"=w1555:errorcluster)  [unwired: 7 in, 2 out]
                    }
                    frame #1 {
                      n637 = call "IV setpotential.vi"("error in (no error)"=w1560, "value"=w1561) -> ("error out"=w1559:errorcluster)  [unwired: 7 in, 2 out]
                    }
                    frame #2 {
                      n638 = call "IV getcurrent.vi"("error in (no error)"=w1563) -> ("error out"=w1562:errorcluster, "value out"=w1564:dbl)  [unwired: 8 in, 1 out]
                      n639 = call "Current ranging routine (SubVI).vi"("Current"=w1564) -> ()  [unwired: 11 in]
                    }
                  }
                }
                frame True {
                  w1573 = 0 items=["Off", "On"] ("CellOnOff")
                  n640 = property on="Ei" class="Ref (strict)"() -> ("Value"=w1565:refnum<k24>)  [unwired: 2 in, 2 out]
                  n641 = disable-structure shown="Enabled" {
                    disable-tunnel: [w1593 _] -> w1571
                    disable-tunnel: [w1592 _] -> w1570
                    disable-tunnel: [w1591 -3 ("range integer")] -> w1569
                    disable-tunnel: w1568 -> [w1589 _]
                    disable-tunnel: w1567 -> [w1587 _]
                    disable-tunnel: w1565 -> [w1582 _]
                    frame Disabled {
                      w1588 = -2 items=["CR07_1A"=0, "CR06_10A"=1, "CR01_100A"=2, "CR00_1000A"=3, "CR05_20A"=20, "CR04_40A"=40, "CR03_50A"=60, "CR02_80A"=80, "CR19_1pA"=-12, "CR18_10pA"=-11, "CR17_100pA"=-10, "CR16_1nA"=-9, "CR15_10nA"=-8, "CR14_100nA"=-7, "CR13_1uA"=-6, "CR12_10uA"=-5, "CR11_100uA"=-4, "CR10_1mA"=-3, "CR09_10mA"=-2, "CR08_100mA"=-1] ("CurrentRange")
                      w1590 = 0 items=["Potentiostatic", "Galvanostatic"] ("Mode")
                      n642 = property class="EI"(reference=w1582, error in=w1587, "Setpoint"=w1589, "Mode"=w1590, "CurrentRange"=w1588) -> (error out=w1584:errorcluster)  [unwired: 1 out]
                      n643 = property on="Sampler 2" class="Ref (strict)"() -> ("Value"=w1583:refnum<k24>)  [unwired: 2 in, 2 out]
                      n644 = property class="EI"(reference=w1582, error in=w1584) -> ("Current"=w1585:dbl, "Potential"=w1586:dbl)  [unwired: 2 out]
                      n645 = property class="EI" props=["EiStatusSupportedFor"](reference=w1582) -> (error out=w1593:errorcluster)  [unwired: 1 in, 2 out]
                      n646 = invoke class="Sampler" method="Sample"(reference=w1583) -> (error out=w1592:errorcluster)  [unwired: 2 in, 2 out]
                      n647 = flat-sequence {
                        tunnel: [w1597] -> w1591
                        tunnel: w1586 -> [w1596]
                        tunnel: w1585 -> [w1595]
                        frame #0 {
                          n648 = Wait (ms)(milliseconds to wait=u32 50) -> ()  [unwired: 1 out]
                        }
                        frame #1 {
                          n649 = call "Range_selector.vi"("potential"=w1596, "current"=w1595) -> ("range integer"=w1597:i32)  [unwired: 9 in]
                        }
                      }
                    }
                    frame Enabled {
                    }
                  }
                  n650 = property class="EI"(reference=w1565, "CellOnOff"=w1573, "CurrentRange"=w1569) -> (error out=w1572:errorcluster)  [unwired: 1 in, 1 out]
                  n651 = disable-structure shown="Enabled" {
                    disable-tunnel: w1572 -> [w1581 _]
                    disable-tunnel: w1571 -> [w1579 _]
                    disable-tunnel: w1570 -> [w1578 _]
                    disable-tunnel: [w1577 _] -> w1566
                    disable-tunnel: w1565 -> [w1576 _]
                    frame Disabled {
                      n652 = call "P_Stat_Status1.vi"("error in (no error)"=w1581, ".NET Refnum in"=w1576) -> ("error out"=w1580:errorcluster, "PotentialOverload"=w1575:bool, "CurrentOverload"=w1574:bool)  [unwired: 3 in, 4 out]
                      n653 = property on="CurrentOverload" class="Bool (strict)"("Value"=w1574) -> ()  [unwired: 2 in, 2 out]
                      n654 = Merge Errors(w1580, w1579, w1578) -> (w1577:errorcluster)
                      n655 = property on="PotentialOverload" class="Bool (strict)"("Value"=w1575) -> ()  [unwired: 2 in, 2 out]
                    }
                    frame Enabled {
                    }
                  }
                }
              }
            }
          }
        }
      }
      frame "Initialse and cool iDus" {
        # "Also re-intialise constants"
        n656 = Unbundle By Name(w1600) -> ("Return detector to \nroom T"=w1603:bool)
        n657 = case shown="True" w1603 {
          tunnel: [State."Wait for Event" ("f") State."Wait for Event" ("f")] -> w1602
          frame False {
            w1612 = 20002  # DRV_SUCCESS
            n658 = stacked-sequence {
              seq-local: [_ _ _ _ _ _ w1678] -> [_ _ _ _ _ _ _]
              seq-local: [_ _ _ _ _ _ w1679] -> [_ _ _ _ _ _ _]
              tunnel: w1612 -> [w1668 _ _ _ _ _ _]
              tunnel: [w1667 _ _ _ _ _ _] -> w1611
              tunnel: [_ _ _ _ _ _ w1678] -> _
              tunnel: [_ _ _ _ _ _ w1679] -> w1606
              frame #0 {
                n659 = call "Initialize.vi"("directory (\"\")"="" ("directory (\"\")")) -> ("DLL error code"=w1670:u32)  [unwired: 1 in, 1 out]
                "Init. return code" <- w1670
                n660 = Equal?(x=w1668, y=w1670) -> (x = y?=w1667:bool)
              }
              frame #1 {
                n661 = Wait (ms)(milliseconds to wait=u32 2000) -> ()  [unwired: 1 out]
              }
              frame #2 {
                w1672 = u16 0  # ReadMode
                n662 = call "SetReadMode.vi"("mode"=w1672) -> ()  [unwired: 1 in, 2 out]
              }
              frame #3 {
                w1673 = u16 1  # AcquisitionMode
                n663 = call "SetAcquisitionMode.vi"("mode"=w1673) -> ()  [unwired: 1 in, 2 out]
              }
              frame #4 {
                w1674 = 0
                n664 = call "SetHSSpeed.vi"("index"=w1674, "type"=w1674) -> ()  [unwired: 2 in, 2 out]
              }
              frame #5 {
                n665 = call "GetNumberVSSpeeds.vi"() -> ("number"=w1677:i32)  [unwired: 3 in, 2 out]
                n666 = Subtract(x=w1677, y=1) -> (x-y=w1675:i32)
                n667 = call "SetVSSpeed.vi"("index"=w1675) -> ()  [unwired: 1 in, 2 out]
              }
              frame #6 {
                n668 = call "GetDetector.vi"() -> ("ypixels"=w1678:i32, "xpixels"=w1679:i32)  [unwired: 4 in, 2 out]
                "xpixels" <- w1679
                "ypixels" <- w1678
              }
            }
            n669 = flat-sequence {
              tunnel: w1611 -> [w1663]
              tunnel: [w1662] -> w1610
              frame #0 {
                n670 = case shown="False" w1663 {
                  selector: w1663 -> [w1665 w1666]
                  tunnel: [w1664 w1666] -> w1662
                  frame False {
                    n671 = Not(x=w1665) -> (.not. x?=w1664:bool)
                    n672 = call "Display Message to User5"() -> ()  [unwired: 10 in, 2 out]
                    n673 = Stop(stop? (T)=w1664) -> ()
                  }
                  frame True {
                  }
                }
              }
            }
            n674 = flat-sequence {
              tunnel: w1610 -> [w1619]
              tunnel: [w1617] -> w1607
              tunnel: w1606 -> [w1617]
              tunnel: [w1616] -> _
              frame #0 {
                w1620 = 36  # DRV_TEMP_STABILIZED
                w1621 = 20002  # DRV_SUCCESS
                # "set T ok?"
                # "timings ok?"
                n675 = stacked-sequence {
                  seq-local: [_ _ w1624 _ _ _] -> [_ _ _ _ _ _]
                  seq-local: [_ _ _ w1632 _ _] -> [_ _ _ _ w1636 w1637]
                  tunnel: w1621 -> [_ _ w1626 w1635 _ _]
                  tunnel: "Temperature\n(degrees C)" -> [_ _ _ w1633 _ _]
                  tunnel: w1620 -> [_ _ _ _ _ w1638]
                  tunnel: w1619 -> [_ _ w1625 _ _ _]
                  tunnel: [_ _ _ _ _ w1637] -> w1616
                  frame #0 {
                    n676 = call "SetTriggerMode.vi"("mode"=TriggerMode_mode_typedef."Internal") -> ()  [unwired: 1 in, 2 out]
                  }
                  frame #1 {
                    n677 = property on="Exposure time (s)" class="DigNum (strict)"() -> ("Value"=w1623:dbl)  [unwired: 2 in, 2 out]
                    n678 = call "SetExposureTime.vi"("time"=w1623) -> ()  [unwired: 1 in, 2 out]
                  }
                  frame #2 {
                    n679 = case shown="True" w1625 {
                      tunnel: w1626 -> [_ w1630]
                      tunnel: [FALSE w1631] -> w1624
                      frame False {
                      }
                      frame True {
                        n680 = call "GetAcquisitionTimings.vi"() -> ("exposure"=→"Calculated exposure time":sgl, "DLL error code"=w1629:u32)  [unwired: 11 in, 3 out]
                        "Check timings return code" <- w1629
                        n681 = Equal?(x=w1630, y=w1629) -> (x = y?=w1631:bool)
                      }
                    }
                  }
                  frame #3 {
                    n682 = call "SetTemperature.vi"("temperature"=w1633) -> ("DLL error code"=w1634:u32)  [unwired: 1 in, 1 out]
                    "Set temprature\nreturn code" <- w1634
                    n683 = Equal?(x=w1635, y=w1634) -> (x = y?=w1632:bool)
                  }
                  frame #4 {
                    n684 = case shown="True" w1636 {
                      frame False {
                      }
                      frame True {
                        n685 = call "CoolerON.vi"() -> ()  [unwired: 2 in, 2 out]
                      }
                    }
                  }
                  frame #5 {
                    n686 = case shown="True" w1637 {
                      tunnel: w1638 -> [_ w1639]
                      frame False {
                      }
                      frame True {
                        n687 = while {
                          tunnel: w1639 -> [w1643]
                          stop <- w1640 continue-if-true
                          n688 = Wait Until Next ms Multiple(millisecond multiple=u32 500) -> ()  [unwired: 1 out]
                          n689 = call "GetTemperature.vi"() -> ("status"=w1641:T18, "temperature"=→"Curent Temp":i32)  [unwired: 4 in, 2 out]
                          n690 = Not Equal?(x=w1643, y=w1641) -> (x != y?=w1640:bool)
                        }
                      }
                    }
                  }
                }
              }
            }
            n691 = for {
              N: 1023 -> [_]
              tunnel: [w1613] -> w1604 mode=indexing
              i -> [w1615]
              n692 = Add(x=1, y=w1615) -> (x+y=w1613:i32)
            }
            n693 = stacked-sequence {
              seq-local: [w1646 _ _] -> [_ w1651 _]
              tunnel: TRUE -> [w1645 _ _]
              tunnel: w1607 -> [_ _ w1660]
              tunnel: w1604 -> [_ _ w1658]
              frame #0 {
                n694 = case shown="True" w1645 {
                  tunnel: [FALSE w1650] -> w1646
                  frame False {
                  }
                  frame True {
                    w1648 = 20002  # DRV_SUCCESS
                    n695 = call "StartAcquisition.vi"() -> ("DLL error code"=w1649:u32)  [unwired: 2 in, 1 out]
                    "Start Aquisition return code" <- w1649
                    n696 = Equal?(x=w1648, y=w1649) -> (x = y?=w1650:bool)
                  }
                }
              }
              frame #1 {
                n697 = case shown="True" w1651 {
                  frame False {
                  }
                  frame True {
                    n698 = while {
                      stop <- w1654 continue-if-true
                      w1653 = u16 72  # DRV ACQUIRING
                      n699 = call "GetStatus.vi"() -> ("status"=w1652:T18)  [unwired: 3 in, 2 out]
                      n700 = Wait Until Next ms Multiple(millisecond multiple=u32 50) -> ()  [unwired: 1 out]
                      n701 = property on="Get status return code" class="DigNum (strict)"("Value"=w1652) -> ()  [unwired: 2 in, 2 out]
                      n702 = Equal?(x=w1652, y=w1653) -> (x = y?=w1654:bool)
                    }
                  }
                }
              }
              frame #2 {
                n703 = call "GetAcquiredData.vi"("size"=w1660) -> ("DLL error code"=→"get aquired data return code":u32, "array"=w1657:i32[])  [unwired: 2 in, 1 out]
                n704 = Bundle(w1658, "array"=w1657) -> (→"?":cluster{i32[], "array":i32[]})  [unwired: 1 in]
                "T reached?" <- TRUE ("T reached?")
              }
            }
          }
          frame True {
            n705 = property on="T reached?" class="Bool (strict)"("Value"=FALSE ("T reached?")) -> ()  [unwired: 2 in, 2 out]
            n706 = stacked-sequence {
              frame #0 {
                n707 = call "CoolerOFF.vi"() -> ("DLL error code"=→"Cooler Off return code":u32)  [unwired: 2 in, 1 out]
              }
              frame #1 {
                n708 = while {
                  stop <- w1685 continue-if-true
                  n709 = call "GetTemperature.vi"() -> ("temperature"=w1683:i32)  [unwired: 4 in, 3 out]
                  n710 = property on="Curent Temp" class="DigNum (strict)"("Value"=w1683) -> ()  [unwired: 2 in, 2 out]
                  n711 = Less?(x=w1683, y=i16 0) -> (x < y?=w1685:bool)
                  n712 = Wait Until Next ms Multiple(millisecond multiple=u32 500) -> ()  [unwired: 1 out]
                }
              }
              frame #2 {
                n713 = call "ShutDown.vi"() -> ()  [unwired: 2 in, 2 out]
                "Shut down sequence run?" <- TRUE ("Shut down complete?")
              }
            }
          }
        }
      }
    }
    n714 = property on="Use autolab?" class="Bool (strict)"() -> ("Value"=w4:bool)  [unwired: 2 in, 2 out]
    n715 = Equal To 0?(x=w22) -> (x = 0?=w30:bool)
    n716 = case shown="True" w4 {
      tunnel: w31 -> [w47 w83]
      tunnel: w30 -> [w46 _]
      tunnel: [w45 w83] -> w24
      tunnel: [w42 FALSE] -> w20
      frame False {
        n717 = case shown="False" w46 {
          tunnel: w47 -> [w56 w82]
          tunnel: [w55 w80] -> w45
          tunnel: [w50 w74] -> w39
          tunnel: [w51 w75] -> w43
          tunnel: [w53 w81] -> w41
          tunnel: [w49 w73] -> w40
          tunnel: [w52 w76] -> w44
          frame False {
            n718 = call "IV getcellstatus.vi"() -> ("devcellstatus out"=w66:i32)  [unwired: 9 in, 2 out]
            n719 = call "Bitget 8-bits test.vi"("x"=w66) -> ("c"=w62:dbl, "e"=w64:dbl, "f"=w63:dbl, "h"=w65:dbl)  [unwired: 19 in, 4 out]
            n720 = Greater?(x=w62, y=0.0) -> (0:w68:bool)
            n721 = Greater?(x=w64, y=0.0) -> (0:w69:bool)
            n722 = Greater?(x=w63, y=0.0) -> (0:w70:bool)
            n723 = Greater?(x=w65, y=0.0) -> (0:w48:bool)
            n724 = And(x=w66, y=256) -> (x .and. y?=w67:i32)
            n725 = Equal?(x=w67, y=256) -> (x = y?=w71:bool)
            n726 = Bundle By Name(cluster=w56, "I overload"=w68, "Aninput1 overload"=w69, "E overload"=w70, "Cell of button pressed"=w48, "Cell on"=w71) -> (w55:T11)
            n727 = Unbundle By Name(w55) -> ("I overload"=w53:bool, "Aninput1 overload"=w52:bool, "E overload"=w51:bool, "Cell of button pressed"=w50:bool, "Cell on"=w49:bool)
          }
          frame True {
            w72 = FALSE
            # "After closing the driver reset the indicators"
            n728 = property class="XYGraph (strict)"("Value"=cluster{dbl[], dbl[]} {[], []} ("XY Graph")) -> ()  [unwired: 2 in, 2 out]
            n729 = property on="Potentiostat Status" class="Str"("Value"="" ("Device Status indicator")) -> ()  [unwired: 2 in, 2 out]
            n730 = property on="Device serial number" class="Str"("Value"="" ("Device serial number")) -> ()  [unwired: 2 in, 2 out]
            n731 = Bundle By Name(cluster=w82, "I overload"=w72, "Aninput1 overload"=w72, "E overload"=w72, "Cell of button pressed"=w72, "Cell on"=w72) -> (w80:T11)
            n732 = Unbundle By Name(w80) -> ("I overload"=w81:bool, "Aninput1 overload"=w76:bool, "E overload"=w75:bool, "Cell of button pressed"=w74:bool, "Cell on"=w73:bool)
          }
        }
        "I_overload" <- w41
        "Aninput1_overload" <- w44
        "E_overload" <- w43
        "cell-off button pressed" <- w39
        "cell on" <- w40
        n733 = Or(x=w41, y=w43) -> (x .or. y?=w42:bool)
      }
      frame True {
      }
    }
    n734 = Unbundle By Name(w31) -> ("Current"=→"current":dbl, "Serial No"=→"Device serial number":string, "Status"=→"Potentiostat Status":string)
    n735 = Or(x=w25, y=w36) -> (x .or. y?=w35:bool)
    n736 = case shown="False" w20 {
      tunnel: w7 -> [w85 w86]
      tunnel: [w85 w86] -> w21
      frame False {
      }
      frame True {
        n737 = disable-structure shown="Disabled" {
          disable-tunnel: [State."Exit" ("f") _] -> _
          frame Disabled {
            n738 = call "Display Message to User"() -> ()  [unwired: 10 in, 2 out]
          }
          frame Enabled {
          }
        }
      }
    }
  }
